vi "Main 2.vi"() -> ()   [LabVIEW 2013]
uses:
  Time_Slot--Control.ctl
  <vilib>/lvdsc/historical/Read Traces (Numeric).vi
  <vilib>/lvdsc/NI_DSC.lvlib
  <vilib>/lvdsc/historical/Read Trace (Numeric).vi
  <userlib>/_OpenG.lib/array/array.llb/Index 1D Array Elements (String)__ogtk.vi
panel:
  in  "Tree":string[](tree)
  out "error out":errorcluster
  out "quality":i32[][](array[numeric])
  in  "options":T1={"interpolate data (F)"=TRUE, "extrapolate to now (F)"=FALSE, "remove data breaks (F)"=TRUE, "interpolation interval (1 s)"=1.0, "maintain trending info (T)"=FALSE} {"interpolation interval (1 s)" min=0.0 format="%0.2f"}
  out "empty?":bool
  out "Argument":string
  in  "Traces":T2(array[cluster])
  out "busy":bool
  out "Array 2":timestamp[](array[timestamp])
  out "Array":timestamp[](array[timestamp])
  out "time (s)":sgl
  out "Children Tags":string[](array[string])
  in  "Presets":u16(ring) items=["Select Preset", "Clear Chart", "Add New Preset"]
  in  "Tab Control":T3(tab)
  in  "Time slots":T4=enum."8 Hours"
  in  "Seek Back Button":bool
  in  "Seek Forward Button":bool
  in  "Display Current":bool
  in  "time interval":T5 {"stop timestamp (now)" format="%<%X\n%x>T"; "start timestamp" format="%<%X\n%x>T"}
  in  "Display Chose Time Slot":bool
  in  "update rate(ms)":i32=10000
  in  "max points per trace (all)":i32=1000
  in  "OK":bool
  out "XY Graph":T6(graph)
  # "Time Window (drop down 1hr 1 day etc)\nchoose channel/s\npresets (inc time window and channels)\nExport to csv.\nLive mode return\nIf you select manual time interval shows that until live mode return button pressed\nwould be nice to have arrows to go back and forth in time."
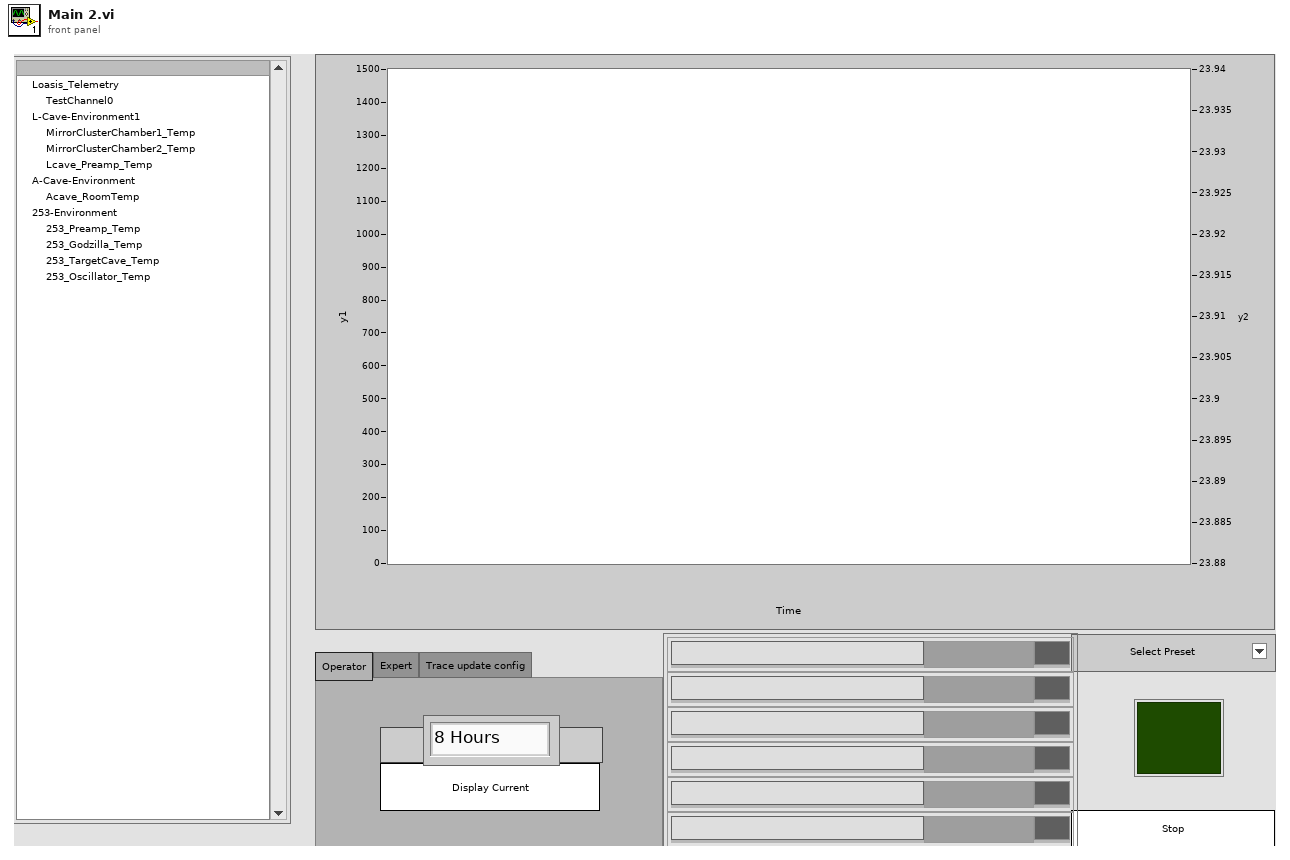
[diagram p1: front panel]
types:
  T1 = cluster{"interpolate data (F)":bool, "extrapolate to now (F)":bool, "remove data breaks (F)":bool, "interpolation interval (1 s)":dbl, "maintain trending info (T)":bool}
  T2 = cluster{"Name":string, "L/R scale":bool, "Color Box":u32}[]
  T3 = enum32{"Operator", "Expert", "Trace update config"}
  T4 = typedef "Time_Slot--Control.ctl" = enum16{"5 Mins", "15 Mins", "30 mins", "1 Hour", "8 Hours", "1 Day", "1 Week", "1 Month", "3 Months", "6 Months", "1 Year", "2 Years"}
  T5 = cluster{"start timestamp":timestamp, "stop timestamp (now)":timestamp}
  T6 = cluster{"timestamps":timestamp[], "data":dbl[]}[]
  T7 = cluster{"Name":string, "L/R scale":bool, "Color Box":u32}
  T8 = enum32{"invalid app kind", "Development System", "Run Time System", "Student Edition", "Embedded LabVIEW", "Evaluation", "Custom"}
  T9 = enum32{"Invalid", "Standard", "Closed", "Hidden", "Minimized", "Maximized"}
  T10 = cluster{"Core":cluster{"Current VI Reference":refnum<vi>, "Close Panel on Exit?":bool}, "options":cluster{"interpolate data (F)":bool, "extrapolate to now (F)":bool, "remove data breaks (F)":bool, "interpolation interval (1 s)":dbl, "maintain trending info (T)":bool}, "time interval":cluster{"start timestamp":timestamp, "stop timestamp (now)":timestamp}, "historical traces":cluster{"timestamps":timestamp[], "data":dbl[]}[], "Trace Names":string[], "max points per trace (all)":i32, "Time slots":T4, "Display Current Enable":bool, "update rate(ms)":i32, "All Traces from DB":string[], "Traces":cluster{"Name":string, "L/R scale":bool, "Color Box":u32}[]}
  T11 = typedef "mysql_authentication.ctl" = cluster{"User":string, "Password":string, "Database":string}
  T12 = cluster{"Port":u16, "IP Address":string, "Authentication":T11}
  T13 = cluster{"Current VI Reference":refnum<vi>, "Close Panel on Exit?":bool}
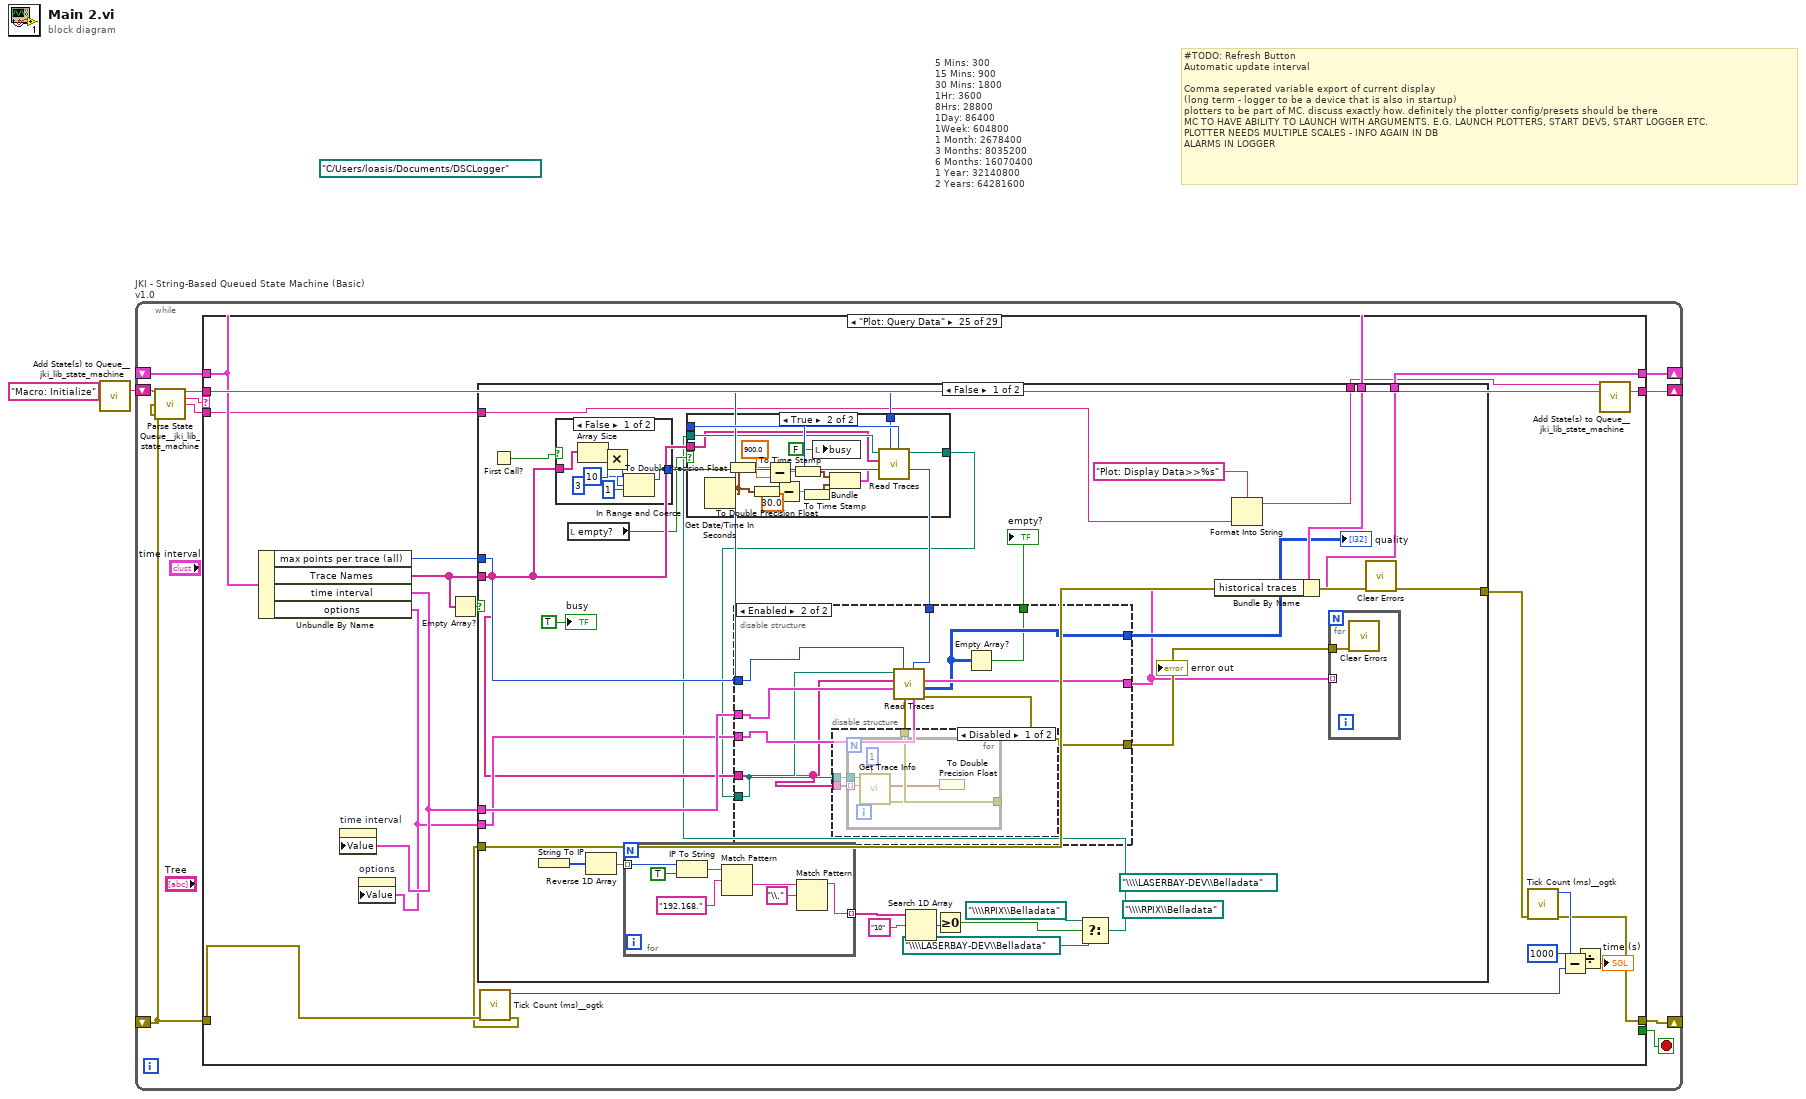
[diagram p0: block diagram]
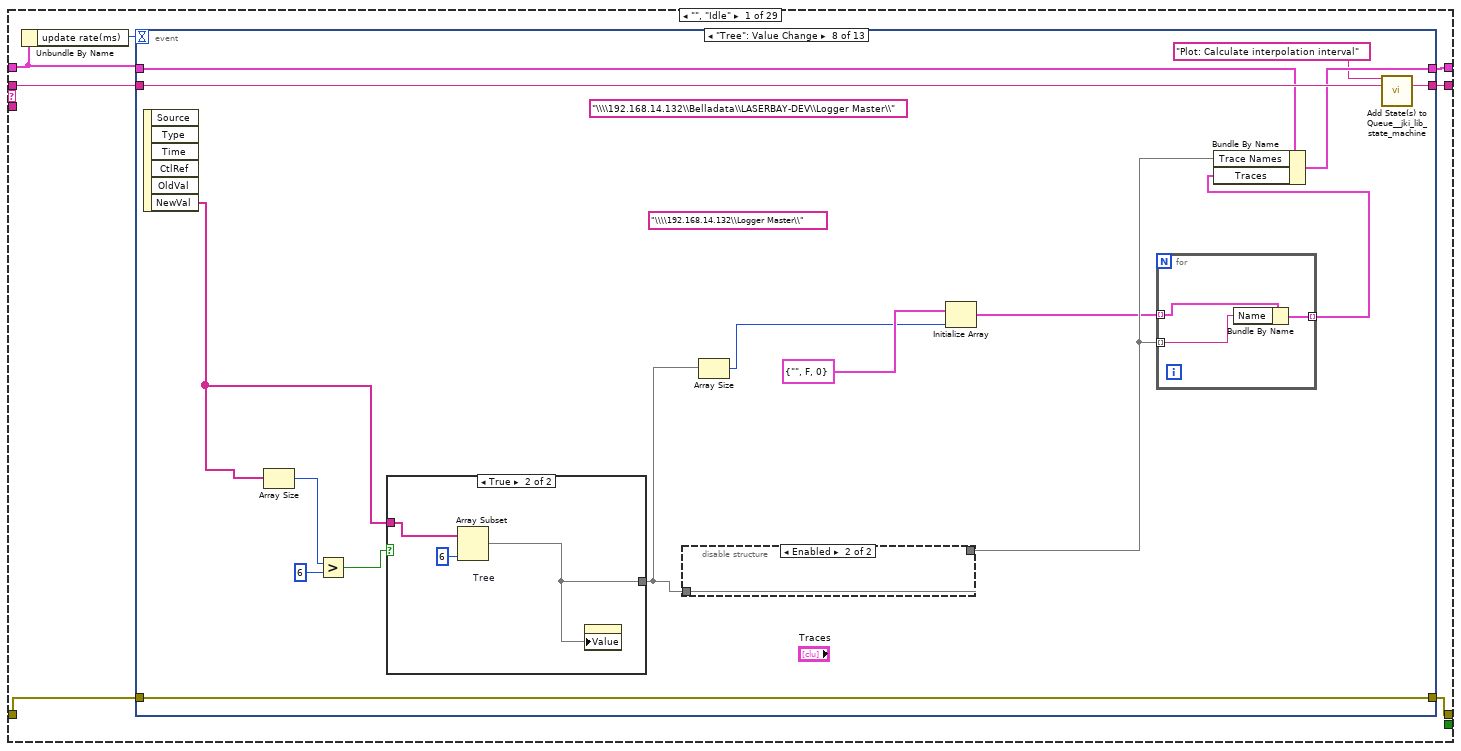
[diagram p2: hidden frame]
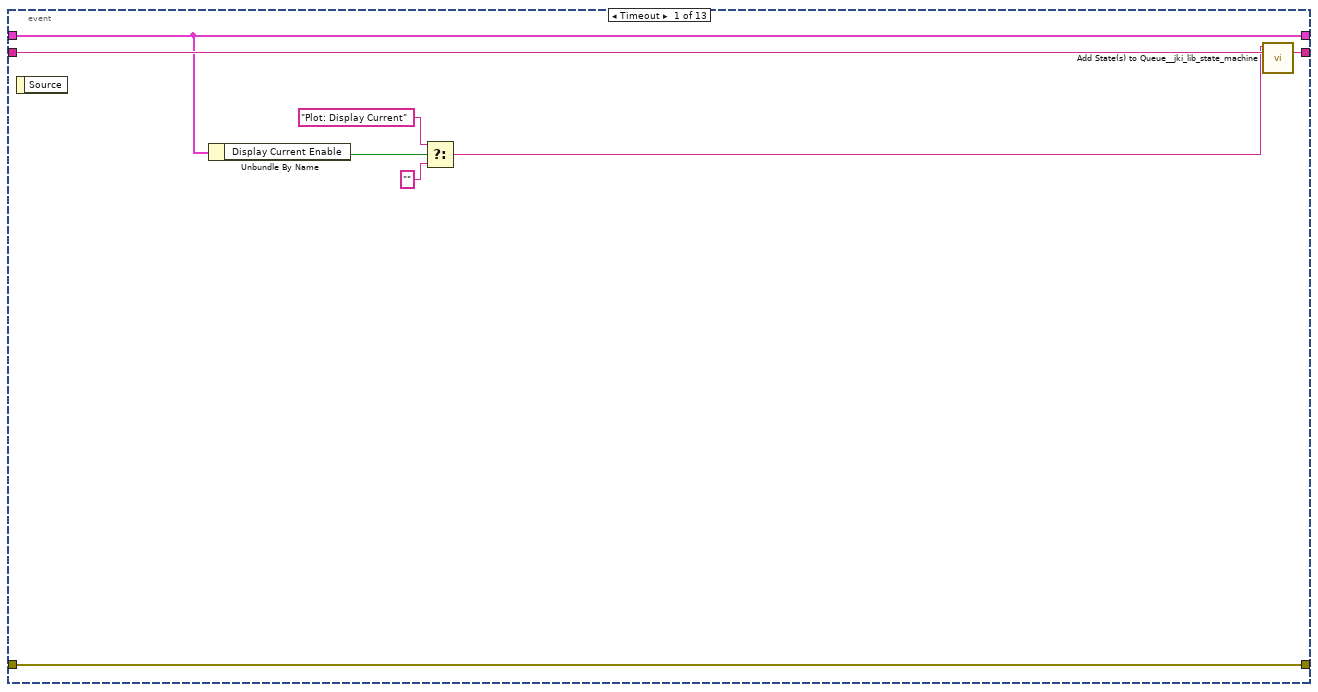
[diagram p3: hidden frame]
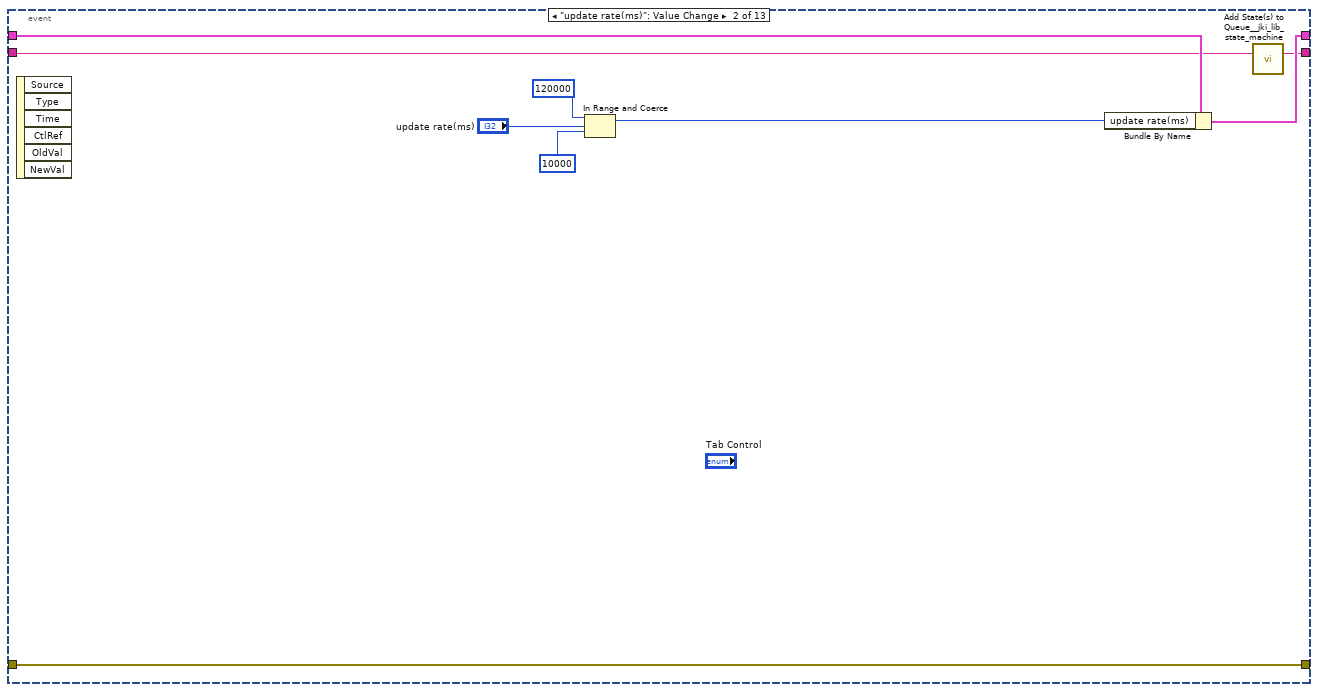
[diagram p4: hidden frame]
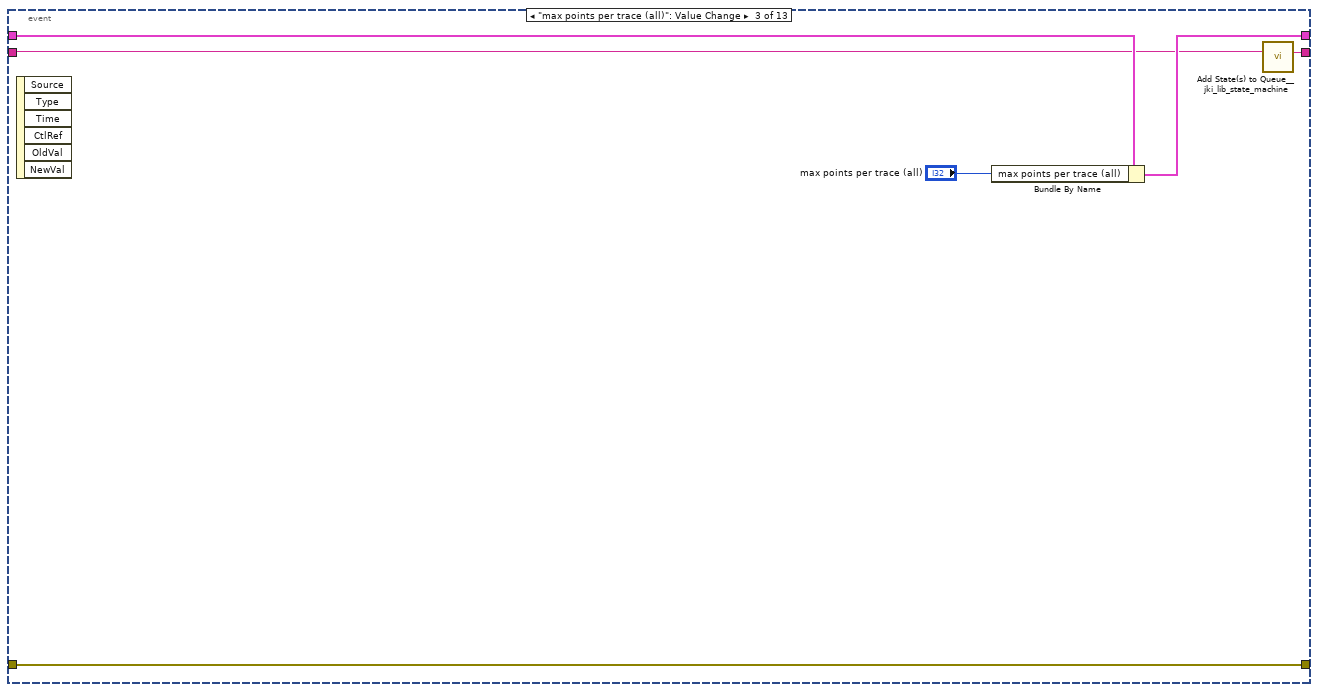
[diagram p5: hidden frame]
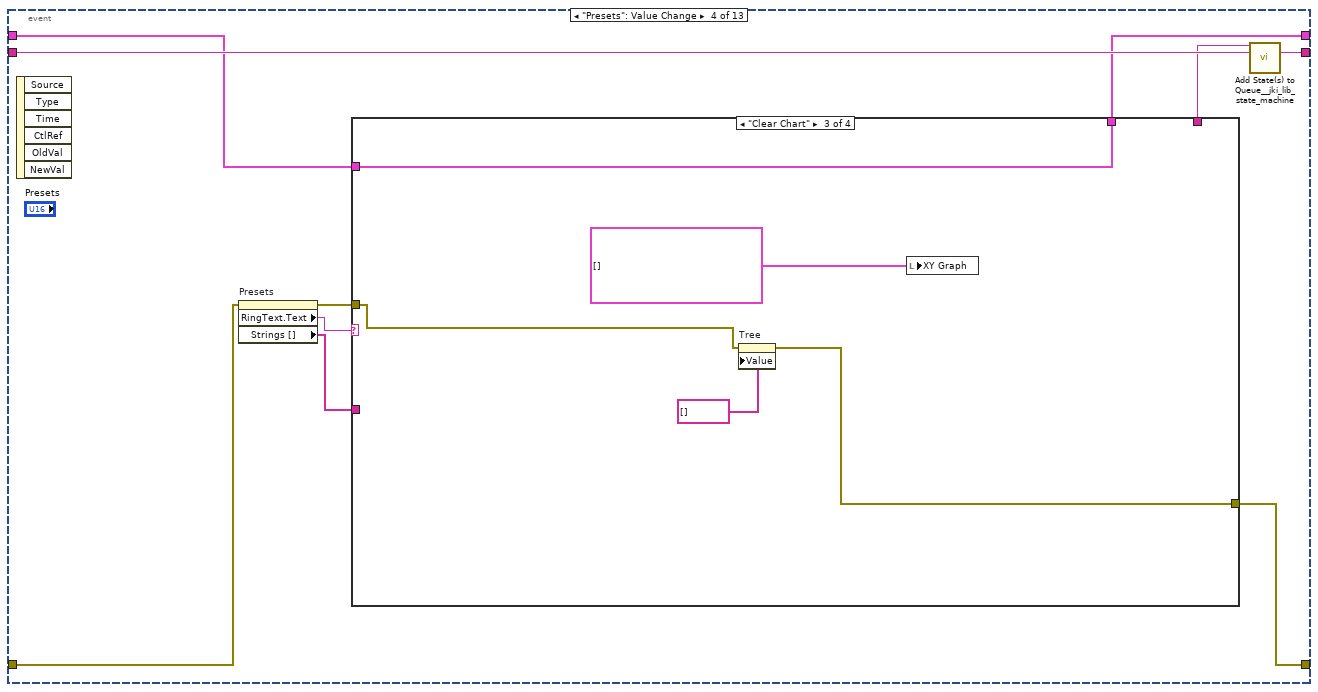
[diagram p6: hidden frame]
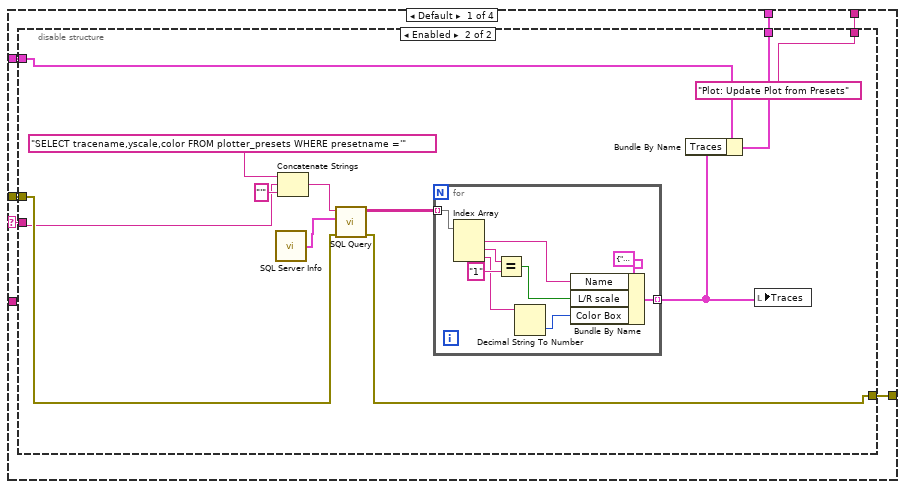
[diagram p7: hidden frame]
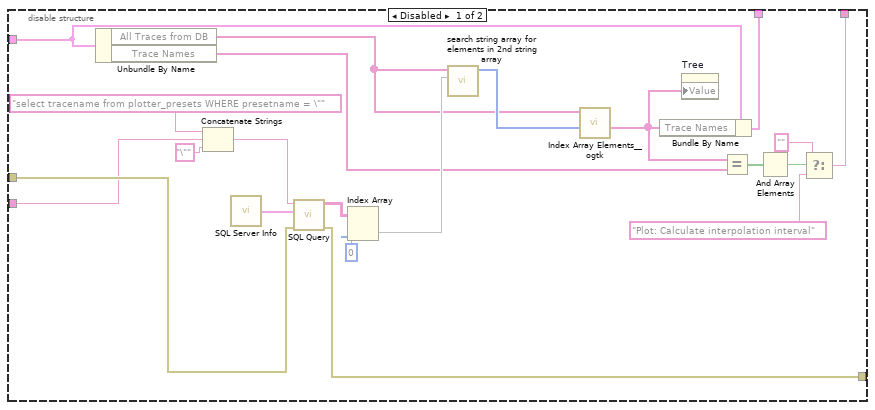
[diagram p8: hidden frame]
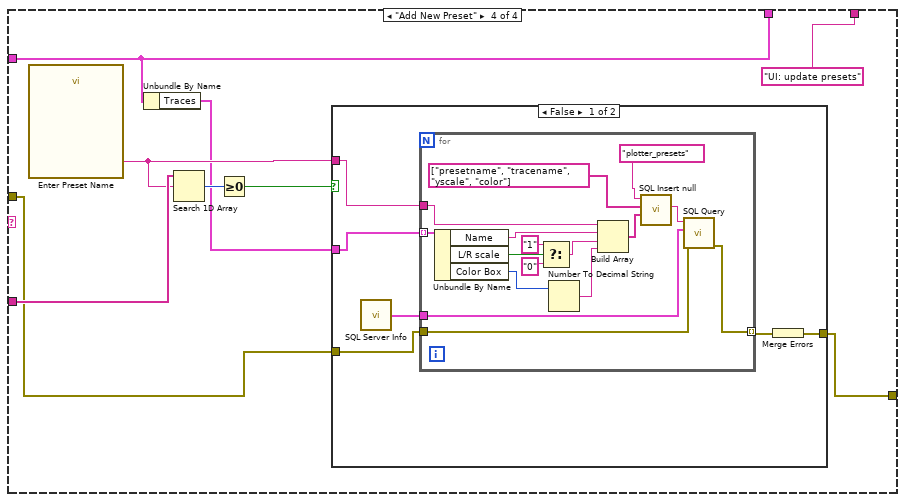
[diagram p10: hidden frame]
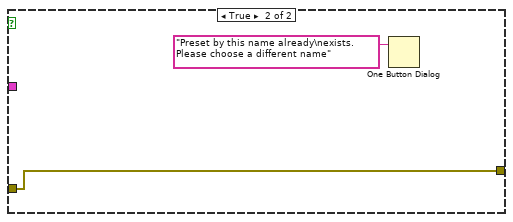
[diagram p11: hidden frame]
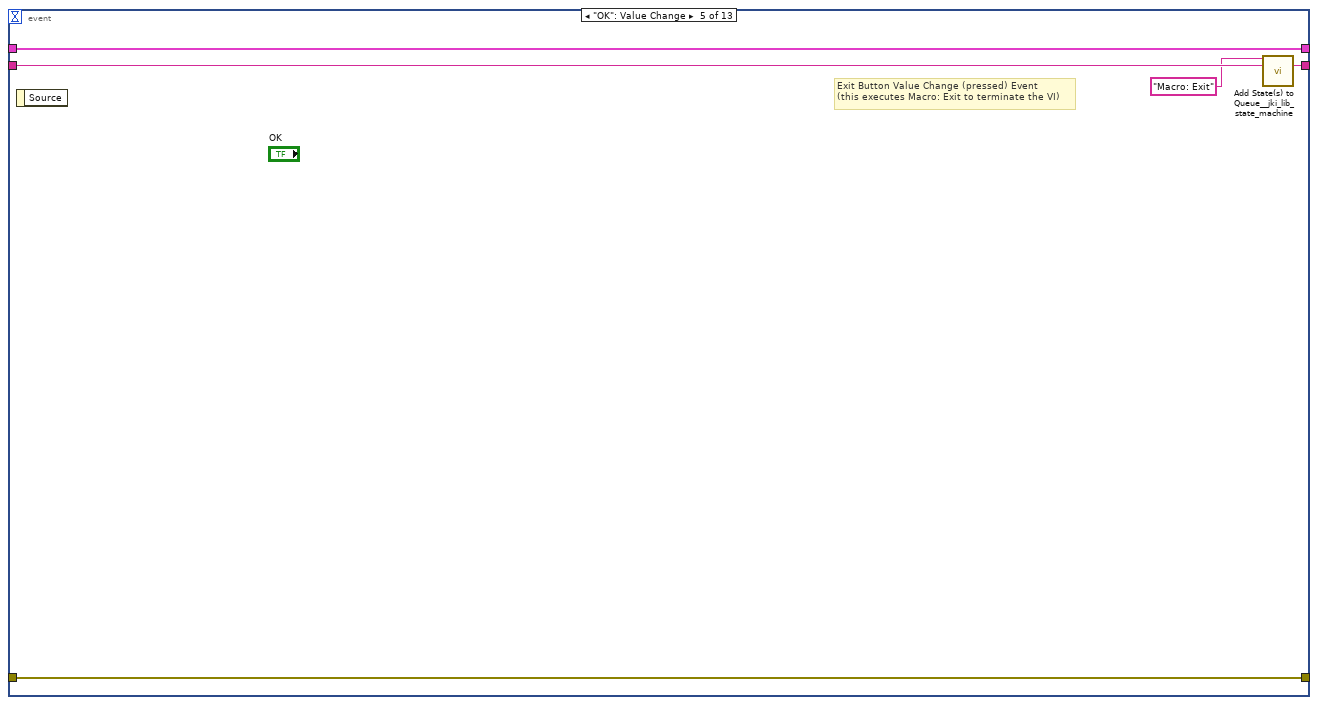
[diagram p12: hidden frame]
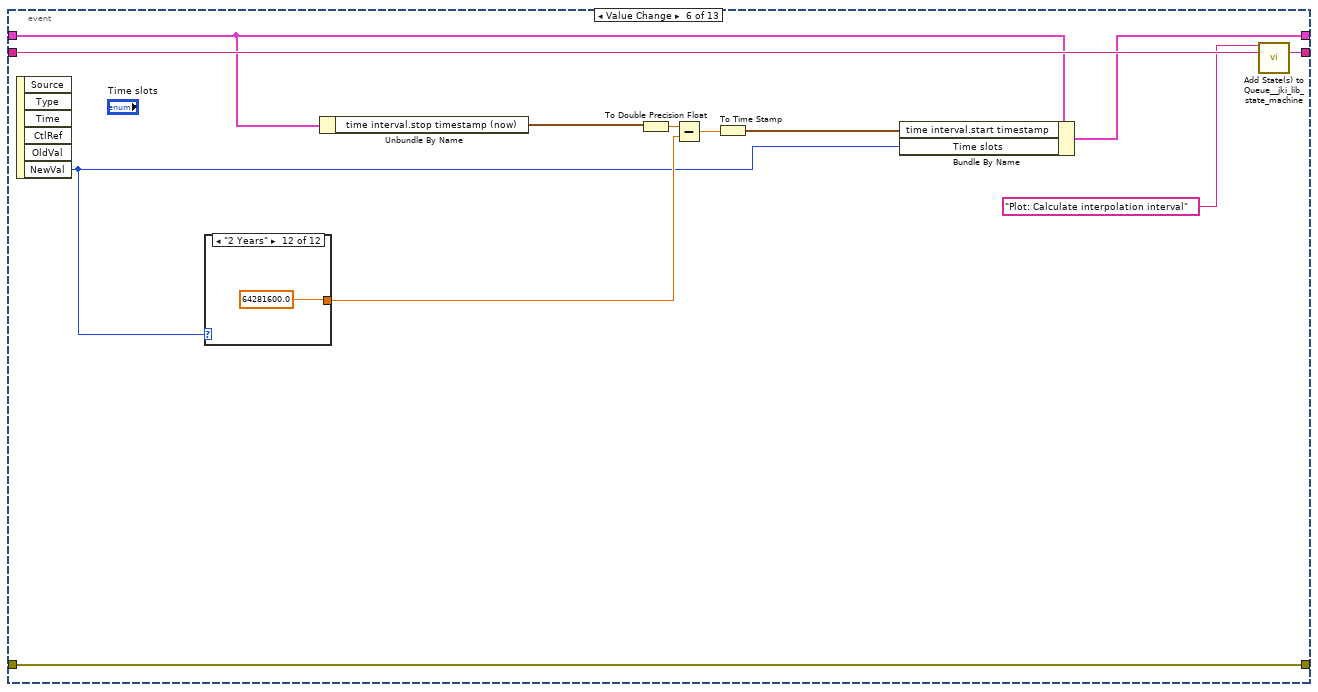
[diagram p13: hidden frame]
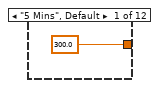
[diagram p14: hidden frame]
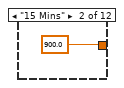
[diagram p15: hidden frame]
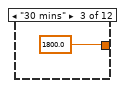
[diagram p16: hidden frame]
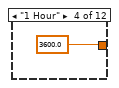
[diagram p17: hidden frame]
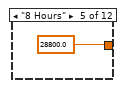
[diagram p18: hidden frame]
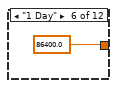
[diagram p19: hidden frame]
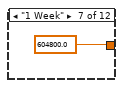
[diagram p20: hidden frame]
diagram:
  (unwired) path "C:/Users/loasis/Documents/DSCLogger" ("Application Directory")
  # "#TODO: Refresh Button\nAutomatic update interval\n\nComma seperated variable export of current display\n(long term - logger to be a device that is also in startup)\nplotters to be part of MC. discuss exactly how. definitely the plotter config/presets should be there\nMC TO HAVE ABILITY TO LAUNCH WITH ARGUMENTS. E.G. LAUNCH PLOTTERS, START DEVS, START LOGGER ETC.\nPLOTTER NEEDS MULTIPLE SCALES - INFO AGAIN IN DB\nALARMS IN LOGGER"
  # "5 Mins: 300\n15 Mins: 900\n30 Mins: 1800\n1Hr: 3600\n8Hrs: 28800\n1Day: 86400\n1Week: 604800\n1 Month: 2678400\n3 Months: 8035200\n6 Months: 16070400 \n1 Year: 32140800\n2 Years: 64281600"
  n1 = call <vilib>:"Add State(s) to Queue__jki_lib_state_machine.vi"("State(s) in (\"\")"="Macro: Initialize") -> ("States Out"=w2:string)  [unwired: 14 in]
  n2 = while "JKI - String-Based Queued State Machine (Basic) v1.0" {
    shift-right: [w5] -> _
    shift-left: _ -> [w4]
    shift-right: [w8] -> _
    shift-left: _ -> [w3]
    shift-right: [w7] -> _
    shift-left: w2 -> [w9]
    stop <- w6 stop-if-true
    n3 = call <vilib>:"Parse State Queue__jki_lib_state_machine.vi"("State Queue"=w9, "Error In (no error)"=w3) -> ("Remaining States"=w11:string, "Current State"=w12:string, "Arguments"=w10:string)  [unwired: 11 in]
    n4 = case shown="\"Plot: Query Data\"" w12 {
      selector: w12 -> [_ _ w346 _ _ _ _ _ _ _ _ _ _ _ _ _ _ _ _ _ _ _ _ _ _ _ _ _ _]
      tunnel: w11 -> [w19 w345 w350 w368 w374 w379 w383 w404 w410 w414 w429 w442 w470 w486 w497 w523 w528 w538 w542 w546 w551 w568 w577 w600 w620 w744 w761 w772 w782]
      tunnel: w10 -> [_ _ _ _ _ _ _ _ _ _ _ _ _ w481 w491 _ _ _ _ _ _ _ _ w587 w601 w738 _ _ _]
      tunnel: w4 -> [w14 w342 w348 w359 w371 w377 w380 _ w405 w411 w427 w440 w472 w484 w493 w520 w525 w535 w539 w543 w548 w564 w573 w593 w616 w742 w759 w770 w777]
      tunnel: [w17 w343 w352 w365 errorcluster {"status"=FALSE, "code"=0, "source"=""} ("error out") w376 w381 w401 w406 w412 w415 w430 w465 w482 w494 w521 w526 w536 w540 w544 w549 w566 w575 w598 w606 w741 w758 w764 w778] -> w8
      tunnel: w3 -> [w16 w343 w351 w365 w370 w376 w381 w401 w407 w412 w416 w431 w466 w483 w495 w521 w526 w536 w540 w544 w549 w566 w575 w598 w610 w741 w758 w765 w774]
      tunnel: [w18 w344 w349 w367 w373 w378 w382 w403 w409 w413 w428 w441 w471 w485 w496 w522 w527 w537 w541 w545 w550 w567 w576 w599 w619 w743 w760 w771 w781] -> w7
      tunnel: [_ _ _ _ _ TRUE _ _ _ _ _ _ _ _ _ _ _ _ _ _ _ _ _ _ _ _ _ _ _] -> w6
      tunnel: [w15 w342 w348 w366 w371 w377 w380 w402 w405 w411 w427 w440 w472 w484 w493 w520 w525 w535 w539 w543 w548 w563 w572 w592 w615 w742 w759 w769 w776] -> w5
      frame "", "Idle" {
        n5 = Unbundle By Name(w14) -> ("update rate(ms)"=w13:i32)
        n6 = event shown="[7] \"Tree\": Value Change" {
          selector: _ -> [_ _ _ _ _ _ _ _ _ _ _ _ _]
          dyn-events: _ -> [_ _ _ _ _ _ _ _ _ _ _ _ _]
          timeout: w13 -> [_ _ _ _ _ _ _ _ _ _ _ _ _]
          tunnel: w19 -> [w27 w28 w37 w47 w145 w155 w172 w188 w207 w250 w283 w312 w341]
          tunnel: [w26 w29 w38 w48 w144 w156 w173 w189 w208 w251 w284 w313 w340] -> w18
          tunnel: w14 -> [w24 w35 w42 w46 w142 w151 w170 w181 w206 w255 w275 w304 w338]
          tunnel: [w25 w30 w39 w49 w143 w157 w174 w190 w209 w248 w285 w314 w339] -> w17
          tunnel: w16 -> [w25 w30 w39 w52 w143 w157 w174 w190 w209 w248 w285 w314 w339]
          tunnel: [w24 w36 w41 w45 w142 w150 w170 w187 w206 w252 w274 w303 w338] -> w15
          event Timeout {
            n7 = event-data() -> ()  [unwired: 1 in, 1 out]
            n8 = Unbundle By Name(w24) -> ("Display Current Enable"=w23:bool)
            n9 = Select(t="Plot: Display Current" ("State(s) in Front (\"\")"), s=w23, f="" ("State(s) in Front (\"\")")) -> (s? t:f=w21:string)
            n10 = call <vilib>:"Add State(s) to Queue__jki_lib_state_machine.vi"("State(s) in Front (\"\")"=w21, "State(s) in (\"\")"=w27) -> ("States Out"=w26:string)  [unwired: 13 in]
          }
          event "update rate(ms)": Value Change {
            n11 = event-data() -> ()  [unwired: 1 in, 6 out]
            n12 = In Range and Coerce(upper limit=120000, x="update rate(ms)", lower limit=10000) -> (coerced(x)=w31:i32)  [unwired: 1 out]
            n13 = Bundle By Name(cluster=w35, "update rate(ms)"=w31) -> (w36:T10)
            n14 = call <vilib>:"Add State(s) to Queue__jki_lib_state_machine.vi"("State(s) in (\"\")"=w28) -> ("States Out"=w29:string)  [unwired: 14 in]
          }
          event "max points per trace (all)": Value Change {
            n15 = event-data() -> ()  [unwired: 1 in, 6 out]
            n16 = Bundle By Name(cluster=w42, "max points per trace (all)"="max points per trace (all)") -> (w41:T10)
            n17 = call <vilib>:"Add State(s) to Queue__jki_lib_state_machine.vi"("State(s) in (\"\")"=w37) -> ("States Out"=w38:string)  [unwired: 14 in]
          }
          event "Presets": Value Change {
            n18 = event-data() -> ()  [unwired: 1 in, 6 out]
            n19 = property on="Presets" class="Ring (strict)"(error in=w52) -> (error out=w50:errorcluster, "RingText.Text"=w51:string, "Strings []"=w43:string[])  [unwired: 1 in, 1 out]
            n20 = case shown="\"Clear Chart\"" w51 {
              selector: w51 -> [w56 _ _ _]
              tunnel: w50 -> [w58 w101 w103 w112]
              tunnel: [w57 w101 w104 w111] -> w49
              tunnel: w46 -> [w55 w102 w107 w110]
              tunnel: [w54 w102 w107 w110] -> w45
              tunnel: [w53 _ _ "UI: update presets" ("t")] -> w44
              tunnel: w43 -> [_ _ _ w116]
              frame Default {
                n21 = disable-structure shown="Enabled" {
                  disable-tunnel: w58 -> [w78 w86]
                  disable-tunnel: [w77 w85] -> w57
                  disable-tunnel: w56 -> [w76 w84]
                  disable-tunnel: w55 -> [w67 w82]
                  disable-tunnel: [w66 w83] -> w54
                  disable-tunnel: [w60 "Plot: Update Plot from Presets" ("t")] -> w53
                  frame Disabled {
                    n22 = Unbundle By Name(w67) -> ("All Traces from DB"=w68:string[], "Trace Names"=w65:string[])
                    n23 = Concatenate Strings("select tracename from plotter_presets WHERE presetname = \"", w76, "\"" ("string")) -> (w74:string)
                    n24 = call "SQL Server Info.vi"() -> ("SQL Server Info"=w79:T12)
                    n25 = call "SQL Query.vi"("error in (no error)"=w78, "SQL Server Info"=w79, "Query"=w74) -> ("error out"=w77:errorcluster, "data"=w72:string[][])  [unwired: 7 in]
                    n26 = Index Array(array=w72, index (col)=0 ("index (row)")) -> (element=w70:string[])  [unwired: 1 in]
                    n27 = call "search string array for elements in 2nd string array.vi"("search for"=w70, "search in"=w68) -> ("Indices of Elements"=w69:i32[])  [unwired: 9 in]
                    n28 = call-poly <userlib>:"Index Array Elements__ogtk.vi"("indices"=w69, "array"=w68) -> ("elements"=w59:string[])  [unwired: 9 in]
                    n29 = Bundle By Name(cluster=w67, "Trace Names"=w59) -> (w66:T10)
                    n30 = property on="Tree" class="Tree (strict)"("Value"=w59) -> ()  [unwired: 2 in, 2 out]
                    n31 = Equal?(x=w59, y=w65) -> (x = y?=w64:bool[])
                    n32 = And Array Elements(Boolean array=w64) -> (logical AND=w63:bool)
                    n33 = Select(t="", s=w63, f="Plot: Calculate interpolation interval") -> (s? t:f=w60:string)
                  }
                  frame Enabled {
                    n34 = call "SQL Server Info.vi"() -> ("SQL Server Info"=w89:T12)
                    n35 = Concatenate Strings("SELECT tracename,yscale,color FROM plotter_presets WHERE presetname ='" ("Query"), w84, "'" ("string")) -> (w91:string)
                    n36 = call "SQL Query.vi"("error in (no error)"=w86, "SQL Server Info"=w89, "Query"=w91) -> ("error out"=w85:errorcluster, "data"=w87:string[][])  [unwired: 7 in]
                    n37 = for {
                      tunnel: w87 -> [w99] mode=indexing
                      tunnel: [w92] -> w81 mode=indexing
                      n38 = Index Array(array=w99) -> (element #1=w98:string, element #2=w97:string, element #3=w93:string)  [unwired: 3 in]
                      n39 = Equal?(x=w97, y="1") -> (x = y?=w95:bool)
                      n40 = Decimal String To Number(string=w93) -> (number=w94:i32)  [unwired: 2 in, 1 out]
                      n41 = Bundle By Name(cluster=T7 {"Name"="", "L/R scale"=FALSE, "Color Box"=0} ("Trace cluster"), "Name"=w98, "L/R scale"=w95, "Color Box"=w94) -> (w92:T7)
                    }
                    n42 = Bundle By Name(cluster=w82, "Traces"=w81) -> (w83:T10)
                    n43 = local write "Traces"(w81) -> ()
                  }
                }
              }
              frame "Select Preset" {
              }
              frame "Clear Chart" {
                n44 = property on="Tree" class="Tree (strict)"(error in=w103, "Value"=string[] [] ("Tree")) -> (error out=w104:errorcluster)  [unwired: 1 in, 1 out]
                n45 = local write "XY Graph"(T6 [] ("XY Graph")) -> ()
              }
              frame "Add New Preset" {
                n46 = call "Enter Preset Name"() -> ("Preset Name"=w113:string)  [unwired: 17 in, 2 out]
                n47 = Unbundle By Name(w110) -> ("Traces"=w109:T2)
                n48 = Search 1D Array(1D array=w116, element=w113) -> (index of element=w115:i32)  [unwired: 1 in]
                n49 = Greater Or Equal To 0?(x=w115) -> (x >= 0?=w114:bool)
                n50 = case shown="False" w114 {
                  tunnel: w109 -> [w121 _]
                  tunnel: w113 -> [w120 _]
                  tunnel: w112 -> [w119 w139]
                  tunnel: [w117 w139] -> w111
                  frame False {
                    n51 = call "SQL Server Info.vi"() -> ("SQL Server Info"=w122:T12)
                    n52 = for {
                      tunnel: w122 -> [w138]
                      tunnel: w121 -> [w130] mode=indexing
                      tunnel: w120 -> [w133]
                      tunnel: w119 -> [w132]
                      tunnel: [w131] -> w118 mode=indexing
                      n53 = Unbundle By Name(w130) -> ("Name"=w129:string, "L/R scale"=w128:bool, "Color Box"=w124:u32)
                      n54 = Select(t="1", s=w128, f="0") -> (s? t:f=w125:string)
                      n55 = Number To Decimal String(number=w124) -> (decimal integer string=w123:string)  [unwired: 1 in]
                      n56 = Build Array(w133, w129, w125, w123) -> (w134:string[])
                      n57 = call "SQL Insert null.vi"("Values"=w134, "Column Names"=string[] ["presetname", "tracename", "yscale", "color"], "Table"="plotter_presets") -> ("Query String"=w137:string)  [unwired: 8 in]
                      n58 = call "SQL Query.vi"("error in (no error)"=w132, "SQL Server Info"=w138, "Query"=w137) -> ("error out"=w131:errorcluster)  [unwired: 7 in, 1 out]
                    }
                    n59 = Merge Errors(w118) -> (w117:errorcluster)
                  }
                  frame True {
                    n60 = One Button Dialog(message="Preset by this name already\nexists. Please choose a different name") -> ()  [unwired: 1 in, 1 out]
                  }
                }
              }
            }
            n61 = call <vilib>:"Add State(s) to Queue__jki_lib_state_machine.vi"("State(s) in Front (\"\")"=w44, "State(s) in (\"\")"=w47) -> ("States Out"=w48:string)  [unwired: 13 in]
          }
          event "OK": Value Change {
            # "Exit Button Value Change (pressed) Event\n(this executes Macro: Exit to terminate the VI)"
            n62 = event-data() -> ()  [unwired: 1 in, 1 out]
            n63 = call <vilib>:"Add State(s) to Queue__jki_lib_state_machine.vi"("State(s) in Front (\"\")"="Macro: Exit", "State(s) in (\"\")"=w145) -> ("States Out"=w144:string)  [unwired: 13 in]
          }
          event Value Change {
            n64 = event-data() -> ("NewVal"=w146:T4)  [unwired: 1 in, 5 out]
            n65 = case shown="\"2 Years\"" w146 {
              tunnel: [300.0 ("y") 900.0 ("y") 1800.0 ("y") 3600.0 ("y") 28800.0 ("y") 86400.0 ("y") 604800.0 ("y") 2678400.0 ("y") 8035200.0 ("y") 16070400.0 ("y") 32140800.0 ("y") 64281600.0 ("y")] -> w152
              frame "5 Mins", Default {
              }
              frame "15 Mins" {
              }
              frame "30 mins" {
              }
              frame "1 Hour" {
              }
              frame "8 Hours" {
              }
              frame "1 Day" {
              }
              frame "1 Week" {
              }
              frame "1 Month" {
              }
              frame "3 Months" {
              }
              frame "6 Months" {
              }
              frame "1 Year" {
              }
              frame "2 Years" {
              }
            }
            n66 = Unbundle By Name(w151) -> ("time interval.stop timestamp (now)"=w153:timestamp)
            n67 = To Double Precision Float(number=w153) -> (double precision float=w154:dbl)
            n68 = Subtract(x=w154, y=w152) -> (x-y=w149:dbl)
            n69 = To Time Stamp(1:w149) -> (0:w148:timestamp)
            n70 = Bundle By Name(cluster=w151, "time interval.start timestamp"=w148, "Time slots"=w146) -> (w150:T10)
            n71 = call <vilib>:"Add State(s) to Queue__jki_lib_state_machine.vi"("State(s) in Front (\"\")"="Plot: Calculate interpolation interval" ("State(s) in Front (\"\")"), "State(s) in (\"\")"=w155) -> ("States Out"=w156:string)  [unwired: 13 in]
          }
          event "Display Current": Value Change {
            n72 = event-data() -> ()  [unwired: 1 in, 6 out]
            n73 = call <vilib>:"Add State(s) to Queue__jki_lib_state_machine.vi"("State(s) in Front (\"\")"="Plot: Display Current" ("State(s) in Front (\"\")"), "State(s) in (\"\")"=w172) -> ("States Out"=w173:string)  [unwired: 13 in]
          }
          event "Tree": Value Change {
            (unwired) "\\\\192.168.14.132\\Belladata\\LASERBAY-DEV\\Logger Master\\"
            (unwired) "\\\\192.168.14.132\\Logger Master\\"
            n74 = event-data() -> ("NewVal"=w182:string[])  [unwired: 1 in, 5 out]
            n75 = Array Size(array=w182) -> (size(s)=w185:i32)
            n76 = Greater?(x=w185, y=6) -> (0:w184:bool)
            n77 = case shown="True" w184 {
              tunnel: w182 -> [w194 w196]
              tunnel: [w194 w195] -> w178
              frame False {
              }
              frame True {
                n78 = Array Subset(array=w196, length=6) -> (w195:string[])  [unwired: 1 in]
                n79 = property on="Tree" class="Tree (strict)"("Value"=w195) -> ()  [unwired: 2 in, 2 out]
              }
            }
            n80 = disable-structure shown="Enabled" {
              disable-tunnel: w178 -> [w199 w202]
              disable-tunnel: [w198 w202] -> w180
              frame Disabled {
                n81 = for {
                  tunnel: w199 -> [w200] mode=indexing
                  tunnel: [w200] -> w198 mode=indexing
                  n82 = Concatenate Strings("\\\\LASERBAY-DEV\\Logger Master\\", w200) -> ()  [unwired: 1 out]
                }
              }
              frame Enabled {
              }
            }
            n83 = Array Size(array=w178) -> (size(s)=w177:i32)
            n84 = Initialize Array(T7 {"Name"="", "L/R scale"=FALSE, "Color Box"=0} ("Trace cluster"), w177) -> (w176:T2)
            n85 = for {
              tunnel: w180 -> [w192] mode=indexing
              tunnel: w176 -> [w193] mode=indexing
              tunnel: [w191] -> w175 mode=indexing
              n86 = Bundle By Name(cluster=w193, "Name"=w192) -> (w191:T7)
            }
            n87 = Bundle By Name(cluster=w181, "Trace Names"=w180, "Traces"=w175) -> (w187:T10)
            n88 = call <vilib>:"Add State(s) to Queue__jki_lib_state_machine.vi"("State(s) in Front (\"\")"="Plot: Calculate interpolation interval" ("State(s) in Front (\"\")"), "State(s) in (\"\")"=w188) -> ("States Out"=w189:string)  [unwired: 13 in]
          }
          event "Traces": Value Change {
            n89 = event-data() -> ("OldVal"=w205:T2, "NewVal"=w204:T2)  [unwired: 1 in, 4 out]
            n90 = for {
              tunnel: w205 -> [w222] mode=indexing
              tunnel: w204 -> [w221] mode=indexing
              tunnel: w204 -> [w213]
              i -> [w212]
              n91 = Unbundle By Name(w221) -> ("Name"=w215:string, "L/R scale"=w219:bool, "Color Box"=w218:u32)
              n92 = Unbundle By Name(w222) -> ("Name"=w216:string, "L/R scale"=w220:bool, "Color Box"=w217:u32)
              n93 = Equal?(x=w217, y=w218) -> (x = y?=w210:bool)
              n94 = Equal?(x=w220, y=w219) -> (x = y?=w214:bool)
              n95 = Equal?(x=w216, y=w215) -> (x = y?=w211:bool)
              n96 = case shown="True" w211 {
                tunnel: w214 -> [_ w226]
                tunnel: w213 -> [_ w225]
                tunnel: w212 -> [_ w224]
                tunnel: w210 -> [_ w223]
                frame False {
                }
                frame True {
                  n97 = stacked-sequence {
                    tunnel: w226 -> [w229 _]
                    tunnel: w225 -> [w228 w240]
                    tunnel: w224 -> [w227 w239]
                    tunnel: w223 -> [_ w241]
                    frame #0 {
                      n98 = case shown="False" w229 {
                        tunnel: w228 -> [w237 _]
                        tunnel: w227 -> [w231 _]
                        frame False {
                          (unwired) u8 2 ("Y Scale.Scale Fit")
                          n99 = Index Array(array=w237, index=w231) -> (element=w236:T7)
                          n100 = Unbundle By Name(w236) -> ("L/R scale"=w235:bool)
                          n101 = To Unsigned Long Integer(number=w231) -> (unsigned 32bit integer=w230:u32)
                          n102 = Select(t=u32 1 ("f"), s=w235, f=u32 0) -> (s? t:f=w233:u32)
                          n103 = control-ref of="XY Graph"() -> (w238:refnum<vi>)
                          n104 = property class="XYGraph (strict)"(reference=w238, "Active Plot"=w230, "Plot.YScaleIdx"=w233) -> ()  [unwired: 1 in, 2 out]
                        }
                        frame True {
                        }
                      }
                    }
                    frame #1 {
                      n105 = case shown="False" w241 {
                        tunnel: w240 -> [w244 _]
                        tunnel: w239 -> [w243 _]
                        frame False {
                          n106 = Index Array(array=w244, index=w243) -> (element=w246:T7)
                          n107 = Unbundle By Name(w246) -> ("Color Box"=w242:u32)
                          n108 = To Unsigned Long Integer(number=w243) -> (unsigned 32bit integer=w245:u32)
                          n109 = control-ref of="XY Graph"() -> (w247:refnum<vi>)
                          n110 = property class="XYGraph (strict)"(reference=w247, "Active Plot"=w245, "Plot.Plot Color"=w242) -> ()  [unwired: 1 in, 2 out]
                        }
                        frame True {
                        }
                      }
                    }
                  }
                }
              }
            }
            n111 = call <vilib>:"Add State(s) to Queue__jki_lib_state_machine.vi"("State(s) in Front (\"\")"="Plot: Display Data" ("State(s) in Front (\"\")"), "State(s) in (\"\")"=w207) -> ("States Out"=w208:string)  [unwired: 13 in]
          }
          event "Display Chose Time Slot": Value Change {
            n112 = event-data() -> ()  [unwired: 1 in, 6 out]
            n113 = property on="time interval" class="Clust (strict)"() -> ("Value"=w261:T5)  [unwired: 2 in, 2 out]
            n114 = Unbundle By Name(w261) -> ("start timestamp"=w254:timestamp, "stop timestamp (now)"=w253:timestamp)
            n115 = To Double Precision Float(number=w254) -> (double precision float=w259:dbl)
            n116 = To Double Precision Float(number=w253) -> (double precision float=w260:dbl)
            n117 = Subtract(x=w259, y=w260) -> (x-y=w258:dbl)
            n118 = Greater?(x=w258, y=60.0) -> (0:w256:bool)
            n119 = case shown="True" w256 {
              tunnel: w255 -> [w263 w268]
              tunnel: w254 -> [_ w267]
              tunnel: w253 -> [_ w266]
              tunnel: [w263 w265] -> w252
              tunnel: ["" "Plot: Calculate interpolation interval" ("State(s) in Front (\"\")")] -> w249
              frame False {
              }
              frame True {
                n120 = Bundle By Name(cluster=w268, "time interval.start timestamp"=w267, "time interval.stop timestamp (now)"=w266) -> (w265:T10)
              }
            }
            n121 = call <vilib>:"Add State(s) to Queue__jki_lib_state_machine.vi"("State(s) in Front (\"\")"=w249, "State(s) in (\"\")"=w250) -> ("States Out"=w251:string)  [unwired: 13 in]
          }
          event "Seek Back Button": Value Change {
            n122 = event-data() -> ()  [unwired: 1 in, 6 out]
            n123 = Unbundle By Name(w275) -> ("Time slots"=w281:T4)
            n124 = case shown="\"15 Mins\"" w281 {
              tunnel: [300.0 ("y") 900.0 ("y") 1800.0 ("y") 3600.0 ("y") 28800.0 ("y") 86400.0 ("y") 604800.0 ("y") 2678400.0 ("y") 8035200.0 ("y") 16070400.0 ("y") 32140800.0 ("y") 64281600.0 ("y")] -> w276
              frame "5 Mins", Default {
              }
              frame "15 Mins" {
              }
              frame "30 mins" {
              }
              frame "1 Hour" {
              }
              frame "8 Hours" {
              }
              frame "1 Day" {
              }
              frame "1 Week" {
              }
              frame "1 Month" {
              }
              frame "3 Months" {
              }
              frame "6 Months" {
              }
              frame "1 Year" {
              }
              frame "2 Years" {
              }
            }
            n125 = Unbundle By Name(w275) -> ("time interval.start timestamp"=w279:timestamp, "time interval.stop timestamp (now)"=w277:timestamp)
            n126 = To Double Precision Float(number=w279) -> (double precision float=w280:dbl)
            n127 = To Double Precision Float(number=w277) -> (double precision float=w278:dbl)
            n128 = Subtract(x=w280, y=w276) -> (x-y=w273:dbl)
            n129 = Subtract(x=w278, y=w276) -> (x-y=w270:dbl)
            n130 = To Time Stamp(1:w273) -> (0:w272:timestamp)
            n131 = To Time Stamp(1:w270) -> (0:w271:timestamp)
            n132 = Bundle By Name(cluster=w275, "time interval.start timestamp"=w272, "time interval.stop timestamp (now)"=w271, "Display Current Enable"=FALSE) -> (w274:T10)
            n133 = call <vilib>:"Add State(s) to Queue__jki_lib_state_machine.vi"("State(s) in Front (\"\")"="Plot: Calculate interpolation interval" ("State(s) in Front (\"\")"), "State(s) in (\"\")"=w283) -> ("States Out"=w284:string)  [unwired: 13 in]
          }
          event "Seek Forward Button": Value Change {
            n134 = event-data() -> ()  [unwired: 1 in, 6 out]
            n135 = Unbundle By Name(w304) -> ("Time slots"=w310:T4)
            n136 = case shown="\"2 Years\"" w310 {
              tunnel: [300.0 ("y") 900.0 ("y") 1800.0 ("y") 3600.0 ("y") 28800.0 ("y") 86400.0 ("y") 604800.0 ("y") 2678400.0 ("y") 8035200.0 ("y") 16070400.0 ("y") 32140800.0 ("y") 64281600.0 ("y")] -> w305
              frame "5 Mins", Default {
              }
              frame "15 Mins" {
              }
              frame "30 mins" {
              }
              frame "1 Hour" {
              }
              frame "8 Hours" {
              }
              frame "1 Day" {
              }
              frame "1 Week" {
              }
              frame "1 Month" {
              }
              frame "3 Months" {
              }
              frame "6 Months" {
              }
              frame "1 Year" {
              }
              frame "2 Years" {
              }
            }
            n137 = Unbundle By Name(w304) -> ("time interval.start timestamp"=w308:timestamp, "time interval.stop timestamp (now)"=w306:timestamp)
            n138 = Get Date/Time In Seconds() -> (seconds since 1Jan1904=w301:timestamp)
            n139 = To Double Precision Float(number=w301) -> (double precision float=w299:dbl)
            n140 = To Double Precision Float(number=w308) -> (double precision float=w309:dbl)
            n141 = To Double Precision Float(number=w306) -> (double precision float=w307:dbl)
            n142 = Add(x=w309, y=w305) -> (x+y=w302:dbl)
            n143 = Add(x=w307, y=w305) -> (x+y=w300:dbl)
            n144 = Greater?(x=w300, y=w299) -> (0:w298:bool)
            n145 = case shown="True" w298 {
              tunnel: ["Plot: Calculate interpolation interval" ("State(s) in Front (\"\")") "Plot: Display Current" ("State(s) in Front (\"\")")] -> w311
              tunnel: w304 -> [w320 w322]
              tunnel: [w319 w322] -> w303
              tunnel: w302 -> [w318 _]
              tunnel: w300 -> [w315 _]
              frame False {
                n146 = To Time Stamp(1:w318) -> (0:w317:timestamp)
                n147 = To Time Stamp(1:w315) -> (0:w316:timestamp)
                n148 = Bundle By Name(cluster=w320, "time interval.start timestamp"=w317, "time interval.stop timestamp (now)"=w316) -> (w319:T10)
              }
              frame True {
              }
            }
            n149 = call <vilib>:"Add State(s) to Queue__jki_lib_state_machine.vi"("State(s) in Front (\"\")"=w311, "State(s) in (\"\")"=w312) -> ("States Out"=w313:string)  [unwired: 13 in]
          }
          event Panel Close? {
            # "Discard the event because we'll close the front panel ourselves in Macro: Exit"
            # "Close Panel button (pressed) Event\n(this executes Macro: Exit to terminate the VI)"
            n150 = event-data() -> ()  [unwired: 1 in, 1 out]
            n151 = event-data("Discard?"=TRUE) -> ()  [unwired: 1 in, 1 out]
            n152 = call <vilib>:"Add State(s) to Queue__jki_lib_state_machine.vi"("State(s) in Front (\"\")"="Macro: Exit", "State(s) in (\"\")"=w341) -> ("States Out"=w340:string)  [unwired: 13 in]
          }
        }
      }
      frame "---------- Core ----------" {
        # "Do not put any code in this frame.\n(it is a separator no-op)"
        n153 = call <vilib>:"Add State(s) to Queue__jki_lib_state_machine.vi"("State(s) in (\"\")"=w345) -> ("States Out"=w344:string)  [unwired: 14 in]
      }
      frame Default {
        w355 = 42 items=["No error", "Argument error", "Memory is full", "Out of zone", "End of file", "File already open", "Generic file I/O error", "File not found", "File permission error", "Disk is full", "Duplicate path", "Too many files open", "System feature not enabled", "Resource file not found", "Cannot add resource", "Resource not found", "Image not found", "Image memory error", "Pen does not exist", "Config type invalid", "Config token not found", "Config parse error", "Config memory error", "Bad external code format", "Bad external code offset", "External code not present", "Null window", "Destroy window error", "Null menu", "Print aborted", "Bad print record", "Print driver error", "Windows error during printing", "Memory error during printing", "Print dialog error", "Generic print error", "Invalid device refnum", "Device not found", "Device parameter error", "Device unit error", "Cannot open device", "Device call aborted", "Generic error", "Cancelled by user", "Object ID too low", "Object ID too high", "Object not in heap", "Unknown heap", "Unknown object (invalid DefProc)", "Unknown object (DefProc not in table)", "Message out of range", "Invalid (null) method", "Unknown message", "Manager call not supported", "Bad address", "Network operation in progress", "Network operation timed out", "Connection is busy", "Network attribute not supported", "Network error", "Address in use", "System out of memory", "Connection aborted", "Connection refused", "Not connected", "Already connected", "Connection closed", "Initialization error (interapplication manager)", "Bad occurrence", "Wait on unbound occurrence handler", "Occurrence queue overflow", "Datalog type conflict", "Unused", "Unrecognized type (interapplication manager)", "Memory corrupt", "Failed to make temporary DLL", "Old CIN version", "Drag socket not found", "Failed to load drop-object", "Failed to register OLE object", "Failed to release OLE object", "Format specifier type mismatch", "Unknown format specifier", "Too few format specifiers", "Too many format specifiers", "Scan failed", "Newer CIN version", "Error converting to variant", "Runtime menu error", "Password tampered", "Variant attribute not found", "Incompatible variant data type", "Event data is not available", "Event Store is not present", "Occurrence is not found", "Event Queue is not created", "Event info is not available", "Refnum passed is NULL", "Error retrieving Class GUID", "Error retrieving CoClass GUID", "Error retrieving TypeLib GUID.", "Bad built application magic bytes.", "Specific driver is different from the specific driver associated with the Logical Name.", "There is no session opened to the class driver.", "Max Error", "MAX - Error with config objects", "MAX - Error loading configuration", "MAX - Group not supported"]
        # "Current State"
        # "Do not delete, rename, or modify this frame.\n(this is used to capture unhandled states and typos)"
        # "Handle mistyped state name (developer tool)"
        n154 = Format Into String(format string="Software Exception: Unhandled State \"%s\"." ("message"), error in=w351, w346) -> (resulting string=w354:string, error out=w353:errorcluster)  [unwired: 1 in]
        n155 = call <vilib>:"Error Cluster From Error Code.vi"("show call chain? (False)"=TRUE, "error in (no error)"=w353, "error message (\"\")"=w354, "error code (0)"=w355) -> ("error out"=w352:errorcluster)  [unwired: 5 in]
        n156 = call <vilib>:"Add State(s) to Queue__jki_lib_state_machine.vi"("State(s) in (\"\")"=w350) -> ("States Out"=w349:string)  [unwired: 14 in]
      }
      frame "Initialize Core Data" {
        # "Do not delete, rename, or modify this frame.\n(this is used to determine panel behavior on exit)"
        # "originally closed?"
        # "exe?"
        # "If panel starts closed or is an EXE, then close it when we exit"
        n157 = property class="VI"() -> ("Front Panel.Open"=w364:bool)  [unwired: 2 in, 2 out]
        n158 = property class="App"() -> ("App.Kind"=w363:T8)  [unwired: 2 in, 2 out]
        n159 = control-ref of="Current VI Reference"() -> (w357:refnum<vi>)
        n160 = Not(x=w364) -> (.not. x?=w361:bool)
        n161 = Equal?(x=w363, y=T8."Run Time System" ("Application:Kind")) -> (x = y?=w360:bool)
        n162 = Or(x=w361, y=w360) -> (x .or. y?=w358:bool)
        n163 = Bundle By Name(cluster=w359, "Core.Current VI Reference"=w357, "Core.Close Panel on Exit?"=w358) -> (w366:T10)
        n164 = call <vilib>:"Add State(s) to Queue__jki_lib_state_machine.vi"("State(s) in (\"\")"=w368) -> ("States Out"=w367:string)  [unwired: 14 in]
      }
      frame "Error Handler" {
        # "Unhandled Error -- Display it"
        # "Handle any errors here.\nYou can also output any states to clean-up after errors occur"
        # "Clear error"
        n165 = call <vilib>:"General Error Handler.vi"("error in (no error)"=w370) -> ()  [unwired: 10 in, 5 out]
        n166 = call <vilib>:"Add State(s) to Queue__jki_lib_state_machine.vi"("State(s) in Front (\"\")"="/* Post Error States", "State(s) in (\"\")"=w374) -> ("States Out"=w373:string)  [unwired: 13 in]
      }
      frame "Exit" {
        # "Do not put any code in this frame.\n(No errors that occur here will be handled.)"
        n167 = call <vilib>:"Add State(s) to Queue__jki_lib_state_machine.vi"("State(s) in (\"\")"=w379) -> ("States Out"=w378:string)  [unwired: 14 in]
      }
      frame "---------- Data ----------" {
        # "Do not put any code in this frame.\n(It is a separator no-op. You can make a copy of this frame to create a new Data frame)"
        n168 = call <vilib>:"Add State(s) to Queue__jki_lib_state_machine.vi"("State(s) in (\"\")"=w383) -> ("States Out"=w382:string)  [unwired: 14 in]
      }
      frame "Data: Initialize" {
        w384 = T2 []  # Traces
        w385 = string[] []  # All Traces from DB
        w386 = 1000  # max points per trace (all)
        w387 = 60000  # update rate(ms)
        w388 = T5 {"start timestamp"=timestamp(0 s since 1904-01-01), "stop timestamp (now)"=timestamp(0 s since 1904-01-01)}  # time interval
        w389 = TRUE  # Display Current Enable
        w390 = Time_Slot--Control."8 Hours"  # Time slots
        w397 = string[] []  # Trace Names
        w398 = T6 []  # historical traces
        w400 = T13 {"Current VI Reference"=refnum, "Close Panel on Exit?"=FALSE}  # Core
        # "8 Hrs"
        n169 = Get Date/Time In Seconds() -> (seconds since 1Jan1904=w393:timestamp)
        n170 = To Double Precision Float(number=w393) -> (double precision float=w395:dbl)
        n171 = Subtract(x=w395, y=28800.0) -> (x-y=w394:dbl)
        n172 = To Time Stamp(1:w394) -> (0:w391:timestamp)
        n173 = Bundle By Name(cluster=w388, "stop timestamp (now)"=w393, "start timestamp"=w391) -> (w396:T5)
        n174 = property on="Time slots" class="Enum (strict)"("Value"=w390) -> ()  [unwired: 2 in, 2 out]
        n175 = Bundle("Core"=w400, "options"="options", "time interval"=w396, "historical traces"=w398, "Trace Names"=w397, "max points per trace (all)"=w386, "Time slots"=w390, "Display Current Enable"=w389, "update rate(ms)"=w387, "All Traces from DB"=w385, "Traces"=w384) -> (w402:T10)  [unwired: 1 in]
        n176 = call <vilib>:"Add State(s) to Queue__jki_lib_state_machine.vi"("State(s) in (\"\")"=w404) -> ("States Out"=w403:string)  [unwired: 14 in]
      }
      frame "Data: Cleanup" {
        # "Cleanup any data and references, here.\n(this is called automatically, by the Macro: Exit)"
        n177 = Unbundle By Name(w405) -> ("Core.Current VI Reference"=w408:refnum<vi>)
        n178 = Close Reference(reference=w408, error in (no error)=w407) -> (error out=w406:errorcluster)
        n179 = call <vilib>:"Add State(s) to Queue__jki_lib_state_machine.vi"("State(s) in (\"\")"=w410) -> ("States Out"=w409:string)  [unwired: 14 in]
      }
      frame "---------- UI ----------" {
        # "Do not put any code in this frame.\n(It is a separator no-op. You can make a copy of this frame to create a new UI frame)"
        n180 = call <vilib>:"Add State(s) to Queue__jki_lib_state_machine.vi"("State(s) in (\"\")"=w414) -> ("States Out"=w413:string)  [unwired: 14 in]
      }
      frame "UI: update presets" {
        # "Do not put any code in this frame.\n(It is a separator no-op. You can make a copy of this frame to create a new UI frame)"
        n181 = call "SQL Server Info.vi"() -> ("SQL Server Info"=w424:T12)
        n182 = call "SQL Query.vi"("error in (no error)"=w416, "SQL Server Info"=w424, "Query"="SELECT DISTINCT presetname FROM plotter_presets") -> ("error out"=w417:errorcluster, "data"=w426:string[][])  [unwired: 7 in]
        n183 = Index Array(array=w426, index (col)=0 ("disabled index (col)")) -> (element=w420:string[])  [unwired: 1 in]
        n184 = Insert Into Array(array=string[] ["Select Preset", "Clear Chart", "Add New Preset"], index=2, new element=w420) -> (w419:string[])
        n185 = property on="Presets" class="Ring (strict)"(error in=w417, "Strings []"=w419, "Value"=0) -> (error out=w415:errorcluster)  [unwired: 1 in, 1 out]
        n186 = call <vilib>:"Add State(s) to Queue__jki_lib_state_machine.vi"("State(s) in (\"\")"=w429) -> ("States Out"=w428:string)  [unwired: 14 in]
      }
      frame "UI: Initialize" {
        # "Initialize the User Interface, here.\n(this is called automatically, by the Macro: Init)"
        n187 = invoke on="Tree" class="Tree (strict)" method="Reinit To Default"() -> (error out=w432:errorcluster)  [unwired: 3 in, 2 out]
        n188 = call "SQL Server Info.vi"() -> ("SQL Server Info"=w439:T12)
        n189 = call "SQL Query.vi"("error in (no error)"=w431, "SQL Server Info"=w439, "Query"="SELECT DISTINCT channel_group FROM logger") -> ("error out"=w430:errorcluster, "data"=w434:string[][])  [unwired: 7 in]
        n190 = invoke on="Tree" class="Tree (strict)" method="Edit Tree Items.Delete"(error in=w432, "Delete Children"=TRUE ("Delete Children?")) -> (error out=w438:errorcluster)  [unwired: 3 in, 4 out]
        n191 = Index Array(array=w434, index (col)=0 ("disabled index (col)")) -> (element=w436:string[])  [unwired: 1 in]
        n192 = for {
          tunnel: w436 -> [w444] mode=indexing
          tunnel: w438 -> [w450]
          tunnel: w439 -> [w449]
          n193 = invoke on="Tree" class="Tree (strict)" method="Edit Tree Items.Add Item"(error in=w450, "Child Position"=-1 ("Child Posn"), "Left Cell"=w444, "Child Only?"=FALSE) -> (error out=w445:errorcluster)  [unwired: 5 in, 8 out]
          n194 = Concatenate Strings("SELECT device,variable,alias FROM logger WHERE channel_group ='" ("Query"), w444, "'" ("string")) -> (w446:string)
          n195 = call "SQL Query.vi"("error in (no error)"=w445, "SQL Server Info"=w449, "Query"=w446) -> ("data"=w443:string[][])  [unwired: 7 in, 1 out]
          n196 = for {
            tunnel: w444 -> [w462]
            tunnel: w443 -> [w461] mode=indexing
            n197 = Index Array(array=w461) -> (element #1=w453:string, element #2=w455:string, element #3=w457:string)  [unwired: 3 in]
            n198 = Empty String/Path?(string/path=w457) -> (empty?=w460:bool)
            n199 = Concatenate Strings(w453, " " ("string"), w455) -> (w456:string)
            n200 = Select(t=w456, s=w460, f=w457) -> (s? t:f=w458:string)
            n201 = invoke on="Tree" class="Tree (strict)" method="Edit Tree Items.Add Item"("Parent Tag"=w462, "Left Cell"=w458, "Child Tag"=w458, "Child Only?"=TRUE) -> ()  [unwired: 5 in, 9 out]
          }
        }
        n202 = call <vilib>:"Add State(s) to Queue__jki_lib_state_machine.vi"("State(s) in (\"\")"=w442) -> ("States Out"=w441:string)  [unwired: 14 in]
      }
      frame "UI: Get Tree Items" {
        n203 = control-ref of="Tree"() -> (w469:refnum<vi>)
        n204 = call "getchildren.vi"("Tree Reference In"=w469) -> ("Children Tags"=w468:string[], "Tree Reference Out"=w467:refnum<vi>)  [unwired: 2 in, 1 out]
        n205 = for {
          tunnel: w468 -> [w478] mode=indexing
          shift-right: [w479] -> _
          shift-left: w467 -> [w480]
          tunnel: w466 -> [w477]
          tunnel: [w476] -> w465
          shift-right: [w474] -> w464
          shift-left: string[] [] -> [w473]
          n206 = call "getchildren.vi"("error in (no error)"=w477, "Parent Tag"=w478, "Tree Reference In"=w480) -> ("error out"=w476:errorcluster, "Children Tags"=w475:string[], "Tree Reference Out"=w479:refnum<vi>)
          n207 = Build Array (concatenate)(w473, w475) -> (w474:string[])
        }
        "Children Tags" <- w464
        n208 = call <vilib>:"Add State(s) to Queue__jki_lib_state_machine.vi"("State(s) in (\"\")"=w470) -> ("States Out"=w471:string)  [unwired: 14 in]
      }
      frame "UI: Cursor Set" {
        # "Argument"
        # "Set and Unset Cursor Busy.\n(Usage: \"UI: Cursor Set >> Busy|Idle\")"
        n209 = case shown="\"Idle\", Default" w481 {
          tunnel: w483 -> [w488 w490]
          tunnel: [w487 w489] -> w482
          frame "Idle", Default {
            n210 = call <vilib>:"Unset Busy.vi"("error in (no error)"=w488) -> ("error out"=w487:errorcluster)  [unwired: 10 in]
          }
          frame "Busy" {
            n211 = call <vilib>:"Set Busy.vi"("error in (no error)"=w490) -> ("error out"=w489:errorcluster)  [unwired: 9 in, 1 out]
          }
        }
        n212 = call <vilib>:"Add State(s) to Queue__jki_lib_state_machine.vi"("State(s) in (\"\")"=w486) -> ("States Out"=w485:string)  [unwired: 14 in]
      }
      frame "UI: Front Panel State" {
        # "Argument"
        # "Set Front Panel Open or Closed\n(Usage: \"UI: Front Panel State >> Open|Close\")"
        n213 = Unbundle By Name(w493) -> ("Core.Current VI Reference"=w492:refnum<vi>)
        n214 = case shown="\"Open\", Default" w491 {
          tunnel: w495 -> [w501 w514]
          tunnel: [w503 w515] -> w494
          tunnel: w492 -> [w502 w512]
          frame "Open", Default {
            n215 = property class="VI"(reference=w502, error in=w501) -> (reference out=w499:refnum<vi>, error out=w500:errorcluster, "Front Panel.Open"=w498:bool)
            n216 = case shown="False" w498 {
              tunnel: [w506 w509] -> w503
              tunnel: w500 -> [w505 w509]
              tunnel: w499 -> [w504 _]
              frame False {
                n217 = invoke class="VI" method="FP.Open"(reference=w504, error in=w505, "Activate"=TRUE, "State"=T9."Standard") -> (error out=w506:errorcluster)  [unwired: 1 in, 4 out]
              }
              frame True {
              }
            }
          }
          frame "Close" {
            n218 = property class="VI"(reference=w512, error in=w514) -> (reference out=w511:refnum<vi>, error out=w513:errorcluster, "Front Panel.Open"=w510:bool)
            n219 = case shown="True" w510 {
              tunnel: [w516 w519] -> w515
              tunnel: w513 -> [w516 w518]
              tunnel: w511 -> [_ w517]
              frame False {
              }
              frame True {
                n220 = invoke class="VI" method="FP.Close"(reference=w517, error in=w518) -> (error out=w519:errorcluster)  [unwired: 1 in, 2 out]
              }
            }
          }
        }
        n221 = call <vilib>:"Add State(s) to Queue__jki_lib_state_machine.vi"("State(s) in (\"\")"=w497) -> ("States Out"=w496:string)  [unwired: 14 in]
      }
      frame "---------- Macro ----------" {
        # "Do not put any code in this frame.\n(It is a separator no-op. You can make a copy of this frame to create a new Macro frame)"
        n222 = call <vilib>:"Add State(s) to Queue__jki_lib_state_machine.vi"("State(s) in (\"\")"=w523) -> ("States Out"=w522:string)  [unwired: 14 in]
      }
      frame "Macro: Initialize" {
        w524 = "Data: Initialize\nInitialize Core Data\nUI: Initialize\nUI: update presets\nUI: Front Panel State >> Open\nUI: Get Tree Items\nMISC: get preset from arguments"  # Data: Initialize Initialize Core Data UI: Initialize UI: update presets UI: Front Panel State >> Open UI: Get Tree Items MISC: get preset from arguments
        # "Initialization Macro\n(This is called once, when the VI starts)"
        n223 = call <vilib>:"Add State(s) to Queue__jki_lib_state_machine.vi"("State(s) in Front (\"\")"=w524, "State(s) in (\"\")"=w528) -> ("States Out"=w527:string)  [unwired: 13 in]
      }
      frame "Macro: Exit" {
        # "Exit Macro\n(This is called once, when the VI exits)"
        n224 = Unbundle By Name(w535) -> ("Core.Close Panel on Exit?"=w534:bool)
        n225 = Select(t="UI: Front Panel State >> Close", s=w534, f="") -> (s? t:f=w531:string)
        n226 = call <vilib>:"Add State(s) to Queue__jki_lib_state_machine.vi"("State(s) in (\"\")"=w531, "State(s) at Back (\"\")"="Data: Cleanup\nExit") -> ("States Out"=w529:string)  [unwired: 13 in]
        n227 = call <vilib>:"Add State(s) to Queue__jki_lib_state_machine.vi"("State(s) in Front (\"\")"=w529, "State(s) in (\"\")"=w538) -> ("States Out"=w537:string)  [unwired: 13 in]
      }
      frame "---------- Data Query ----------" {
        # "Template Separator\n(You can make a copy of, or modify, this frame)"
        n228 = call <vilib>:"Add State(s) to Queue__jki_lib_state_machine.vi"("State(s) in (\"\")"=w542) -> ("States Out"=w541:string)  [unwired: 14 in]
      }
      frame "----------------Traces----------------" {
        # "Template Separator\n(You can make a copy of, or modify, this frame)"
        n229 = call <vilib>:"Add State(s) to Queue__jki_lib_state_machine.vi"("State(s) in (\"\")"=w546) -> ("States Out"=w545:string)  [unwired: 14 in]
      }
      frame "MISC: get preset from arguments" {
        # "Template Separator\n(You can make a copy of, or modify, this frame)"
        n230 = disable-structure "Factory Pattern: Enable plugin" shown="RUN_TIME_ENGINE==True" {
          disable-tunnel: [_ ""] -> w547
          frame condition #0 (active) {
          }
          frame condition #1 {
            n231 = control-ref of="This Application"() -> (w559:refnum<vi>)
            n232 = property class="App"(reference=w559) -> ("App.Args"=w557:string[])  [unwired: 1 in, 2 out]
            n233 = Index Array(array=w557, index=1) -> (element=w554:string)
            "Argument" <- w554
            n234 = property on="Presets" class="Ring (strict)"() -> ("Strings []"=w555:string[])  [unwired: 2 in, 2 out]
            n235 = Search 1D Array(1D array=w555, element=w554) -> (index of element=w553:i32)  [unwired: 1 in]
            n236 = Greater Or Equal To 0?(x=w553) -> (x >= 0?=w552:bool)
            n237 = case shown="True" w552 {
              tunnel: w553 -> [_ w560]
              frame False {
              }
              frame True {
                n238 = property on="Presets" class="Ring (strict)"("Val(Sgnl)"=w560) -> ()  [unwired: 2 in, 2 out]
              }
            }
          }
        }
        n239 = call <vilib>:"Add State(s) to Queue__jki_lib_state_machine.vi"("State(s) in Front (\"\")"=w547, "State(s) in (\"\")"=w551) -> ("States Out"=w550:string)  [unwired: 13 in]
      }
      frame "Plot: Update Plot from Presets" {
        n240 = Unbundle By Name(w564) -> ("Traces"=w565:T2)
        n241 = for {
          tunnel: w565 -> [w570] mode=indexing
          tunnel: [w569] -> w561 mode=indexing
          n242 = Unbundle By Name(w570) -> ("Name"=w569:string)
        }
        n243 = property on="Tree" class="Tree (strict)"("Value"=w561) -> ()  [unwired: 2 in, 2 out]
        n244 = Bundle By Name(cluster=w564, "Trace Names"=w561) -> (w563:T10)
        n245 = call <vilib>:"Add State(s) to Queue__jki_lib_state_machine.vi"("State(s) in Front (\"\")"="Plot: Calculate interpolation interval>>preset" ("State(s) in Front (\"\")"), "State(s) in (\"\")"=w568) -> ("States Out"=w567:string)  [unwired: 13 in]
      }
      frame "Traces: update cluster" {
        # "Template Separator\n(You can make a copy of, or modify, this frame)"
        n246 = Unbundle By Name(w573) -> ("Traces"=w574:T2)
        n247 = for {
          tunnel: w574 -> [w581] mode=indexing
          tunnel: [w578] -> w571 mode=indexing
          i -> [w583]
          n248 = control-ref of="XY Graph"() -> (w584:refnum<vi>)
          n249 = property class="XYGraph (strict)"(reference=w584, "Active Plot"=w583) -> ("Plot.YScaleIdx"=w582:u32, "Plot.Plot Color"=w579:u32)  [unwired: 1 in, 2 out]
          n250 = Not Equal To 0?(x=w582) -> (x != 0?=w580:bool)
          n251 = Bundle By Name(cluster=w581, "L/R scale"=w580, "Color Box"=w579) -> (w578:T7)
        }
        n252 = Bundle By Name(cluster=w573, "Traces"=w571) -> (w572:T10)
        n253 = local write "Traces"(w571) -> ()
        n254 = call <vilib>:"Add State(s) to Queue__jki_lib_state_machine.vi"("State(s) in (\"\")"=w577) -> ("States Out"=w576:string)  [unwired: 14 in]
      }
      frame "Plot: Calculate interpolation interval" {
        n255 = Unbundle By Name(w593) -> ("time interval.stop timestamp (now)"=w595:timestamp, "time interval.start timestamp"=w594:timestamp, "max points per trace (all)"=w590:i32)
        n256 = To Double Precision Float(number=w595) -> (double precision float=w596:dbl)
        n257 = To Double Precision Float(number=w594) -> (double precision float=w597:dbl)
        n258 = Subtract(x=w596, y=w597) -> (x-y=w591:dbl)
        n259 = Divide(x=w591, y=w590) -> (x/y=w589:dbl)
        n260 = Format Into String(format string="Plot: Query Data>>%s", w587) -> (resulting string=w585:string)  [unwired: 2 in, 1 out]
        n261 = Round To Nearest(number=w589) -> (nearest integer value=w588:dbl)
        n262 = Bundle By Name(cluster=w593, "options.interpolation interval (1 s)"=w588) -> (w592:T10)
        n263 = call <vilib>:"Add State(s) to Queue__jki_lib_state_machine.vi"("State(s) in Front (\"\")"=w585, "State(s) in (\"\")"=w600) -> ("States Out"=w599:string)  [unwired: 13 in]
      }
      frame "Plot: Query Data" {
        n264 = Unbundle By Name(w616) -> ("max points per trace (all)"=w614:i32, "Trace Names"=w617:string[], "time interval"=w612:T5, "options"=w611:T1)
        n265 = property on="time interval" class="Clust (strict)"("Value"=w612) -> ()  [unwired: 2 in, 2 out]
        n266 = property on="options" class="Clust (strict)"("Value"=w611) -> ()  [unwired: 2 in, 2 out]
        n267 = Empty Array?(array=w617) -> (empty?=w618:bool)
        n268 = call <userlib>:"Tick Count (ms)__ogtk.vi"("error in (no error)"=w610) -> ("error out"=w609:errorcluster, "millisecond timer value"=w605:u32)  [unwired: 9 in]
        n269 = case shown="False" w618 {
          tunnel: w617 -> [w636 _]
          tunnel: w612 -> [w645 _]
          tunnel: w609 -> [w649 w734]
          tunnel: [w646 w734] -> w608
          tunnel: w611 -> [w644 _]
          tunnel: w616 -> [w648 w735]
          tunnel: [w647 w735] -> w615
          tunnel: w614 -> [w637 _]
          tunnel: [w630 _] -> w613
          tunnel: w601 -> [w631 _]
          frame False {
            (unwired) path "\\\\LASERBAY-DEV\\Belladata" ("database URL")
            (unwired) path "\\\\RPIX\\Belladata" ("database URL")
            n270 = First Call?() -> (First Call?: T/F=w641:bool)
            n271 = String To IP() -> (0:w622:u32[])  [unwired: 1 in]
            n272 = case shown="False" w641 {
              tunnel: [w725 30 ("timeout (30 s)")] -> w638
              tunnel: w636 -> [w731 _]
              frame False {
                n273 = Array Size(array=w731) -> (size(s)=w730:i32)
                n274 = Multiply(x=w730, y=3 ("timeout (30 s)")) -> (x*y=w728:i32)
                n275 = In Range and Coerce(upper limit=10, x=w728, lower limit=1) -> (coerced(x)=w725:i32)  [unwired: 1 out]
              }
              frame True {
              }
            }
            n276 = local read "empty?"() -> (w634:bool)
            n277 = Reverse 1D Array(array=w622) -> (reversed array=w623:u32[])
            n278 = for {
              tunnel: w623 -> [w650] mode=indexing
              tunnel: [w651] -> w626 mode=indexing
              n279 = IP To String(1:TRUE ("dot notation? (F)"), 2:w650) -> (0:w652:string)
              n280 = Match Pattern(string=w652, regular expression="192.168.") -> (after substring=w654:string)  [unwired: 1 in, 3 out]
              n281 = Match Pattern(string=w654, regular expression="\\.") -> (before substring=w651:string)  [unwired: 1 in, 3 out]
            }
            n282 = Search 1D Array(1D array=w626, element="10") -> (index of element=w628:i32)  [unwired: 1 in]
            n283 = Greater Or Equal To 0?(x=w628) -> (x >= 0?=w629:bool)
            n284 = Select(t=path "\\\\RPIX\\Belladata" ("Application Directory"), s=w629, f=path "\\\\LASERBAY-DEV\\Belladata" ("Application Directory")) -> (s? t:f=w621:path)
            n285 = case shown="True" w634 {
              tunnel: w621 -> [w657 w668]
              tunnel: w636 -> [_ w667]
              tunnel: w638 -> [_ w666]
              tunnel: w637 -> [_ w665]
              tunnel: [w657 w658] -> w633
              frame False {
              }
              frame True {
                n286 = Get Date/Time In Seconds() -> (seconds since 1Jan1904=w661:timestamp)
                n287 = To Double Precision Float(number=w661) -> (double precision float=w662:dbl)
                n288 = To Double Precision Float(number=w661) -> (double precision float=w664:dbl)
                n289 = Subtract(x=w662, y=900.0) -> (x-y=w671:dbl)
                n290 = Subtract(x=w664, y=30.0) -> (x-y=w660:dbl)
                n291 = To Time Stamp(1:w671) -> (0:w673:timestamp)
                n292 = To Time Stamp(1:w660) -> (0:w659:timestamp)
                n293 = local write "busy"(FALSE ("busy")) -> ()
                n294 = Bundle(w673, w659) -> (w669:cluster{timestamp, timestamp})  [unwired: 1 in]
                n295 = call-poly <vilib>:"Read Traces.vi"("timeout (30 s)"=w666, "max points per trace (all)"=w665, "time interval"=w669, "trace names"=w667, "database URL"=w668) -> ("database URL out"=w658:path)  [unwired: 3 in, 3 out]
              }
            }
            n296 = disable-structure shown="Enabled" {
              disable-tunnel: w636 -> [w685 w709]
              disable-tunnel: w633 -> [w684 w710]
              disable-tunnel: w645 -> [w683 w716]
              disable-tunnel: w644 -> [w682 w714]
              disable-tunnel: w637 -> [w681 w713]
              disable-tunnel: [w680 w707] -> w643
              disable-tunnel: [w678 w715] -> w642
              disable-tunnel: w638 -> [w677 w712]
              disable-tunnel: [w676 w711] -> w639
              disable-tunnel: [_ w706] -> w635
              frame Disabled {
                n297 = for {
                  tunnel: w685 -> [w693] mode=indexing
                  tunnel: w684 -> [w697]
                  tunnel: w683 -> [w695]
                  tunnel: w682 -> [w694]
                  tunnel: [w692] -> w676 mode=indexing
                  tunnel: [w691] -> w680 mode=indexing
                  tunnel: w681 -> [w686]
                  workers-P: 8 -> [_]
                  tunnel: [w690] -> w678
                  tunnel: w677 -> [w689]
                  tunnel: [w688] -> w674 mode=indexing
                  tunnel: [w687] -> w675 mode=indexing
                  n298 = disable-structure shown="Enabled" {
                    disable-tunnel: w697 -> [w704 w705]
                    disable-tunnel: [w702 _] -> w688
                    disable-tunnel: [w701 _] -> w687
                    disable-tunnel: [w700 w705] -> w696
                    disable-tunnel: w693 -> [w699 _]
                    frame Enabled {
                      n299 = call <vilib>:"Get Trace Info.vi"("timeout (30 s)"=5, "trace name"=w699, "database URL"=w704) -> ("error out"=w698:errorcluster, "last timestamp"=w701:timestamp, "first timestamp"=w702:timestamp, "database URL out"=w700:path)  [unwired: 4 in, 1 out]
                      n300 = call <vilib>:"Clear Errors.vi"("error in (no error)"=w698) -> ()  [unwired: 6 in, 1 out]
                    }
                    frame Disabled {
                    }
                  }
                  n301 = call-poly <vilib>:"Read Trace.vi"("options"=w694, "timeout (30 s)"=w689, "max points per trace (all)"=w686, "time interval"=w695, "trace name"=w693, "database URL"=w696) -> ("error out"=w690:errorcluster, "quality"=w691:i32[], "historical trace"=w692:cluster{"timestamps":timestamp[], "data":dbl[]})  [unwired: 2 in, 1 out]
                }
                "Array 2" <- w675
                "Array" <- w674
              }
              frame Enabled {
                n302 = disable-structure shown="Disabled" {
                  disable-tunnel: w710 -> [w719 _]
                  disable-tunnel: w709 -> [w718 _]
                  disable-tunnel: [w717 _] -> w708
                  frame Disabled {
                    n303 = for {
                      tunnel: w719 -> [w724]
                      tunnel: w718 -> [w722] mode=indexing
                      tunnel: [w721] -> w717
                      n304 = call <vilib>:"Get Trace Info.vi"("timeout (30 s)"=1, "trace name"=w722, "database URL"=w724) -> ("error out"=w721:errorcluster, "first timestamp"=w720:timestamp)  [unwired: 4 in, 3 out]
                      n305 = To Double Precision Float(number=w720) -> ()  [unwired: 1 out]
                    }
                  }
                  frame Enabled {
                  }
                }
                n306 = call-poly <vilib>:"Read Traces.vi"("options"=w714, "timeout (30 s)"=w712, "max points per trace (all)"=w713, "error in (no error)"=w708, "time interval"=w716, "trace names"=w709, "database URL"=w710) -> ("error out"=w715:errorcluster, "quality"=w707:i32[][], "historical traces"=w711:T6)  [unwired: 1 in, 1 out]
                n307 = Empty Array?(array=w707) -> (empty?=w706:bool)
              }
            }
            "quality" <- w643
            "error out" <- w642
            "empty?" <- w635
            n308 = Bundle By Name(cluster=w648, "historical traces"=w639) -> (w647:T10)
            n309 = Format Into String(format string="Plot: Display Data>>%s", w631) -> (resulting string=w630:string)  [unwired: 2 in, 1 out]
            n310 = for {
              tunnel: w642 -> [w733]
              tunnel: w639 -> [_] mode=indexing
              n311 = call <vilib>:"Clear Errors.vi"("error in (no error)"=w733) -> ()  [unwired: 6 in, 1 out]
            }
            n312 = call <vilib>:"Clear Errors.vi"("error in (no error)"=w649) -> ("error out"=w646:errorcluster)  [unwired: 6 in]
            "busy" <- TRUE ("Boolean")
          }
          frame True {
          }
        }
        n313 = call <userlib>:"Tick Count (ms)__ogtk.vi"("error in (no error)"=w608) -> ("error out"=w606:errorcluster, "millisecond timer value"=w607:u32)  [unwired: 9 in]
        n314 = Subtract(x=w607, y=w605) -> (x-y=w604:u32)
        n315 = Divide(x=w604, y=u32 1000 ("x")) -> (x/y=→"time (s)":dbl)
        n316 = call <vilib>:"Add State(s) to Queue__jki_lib_state_machine.vi"("State(s) in Front (\"\")"=w613, "State(s) in (\"\")"=w620) -> ("States Out"=w619:string)  [unwired: 13 in]
      }
      frame "Plot: Display Data" {
        n317 = Unbundle By Name(w742) -> ("historical traces"=→"XY Graph":T6, "Traces"=w737:T2)
        n318 = local write "busy"(FALSE ("Boolean")) -> ()
        n319 = case shown="\"preset\"" w738 {
          tunnel: w737 -> [_ w746]
          tunnel: ["Traces: update cluster" ("State(s) in Front (\"\")") "" ("State(s) in Front (\"\")")] -> w736
          frame "False", Default {
          }
          frame "preset" {
            n320 = for {
              tunnel: w746 -> [w751] mode=indexing
              i -> [w752]
              (unwired) u8 2 ("Y Scale.Scale Fit")
              n321 = control-ref of="XY Graph"() -> (w753:refnum<vi>)
              n322 = Unbundle By Name(w751) -> ("L/R scale"=w757:bool, "Color Box"=w750:u32)
              n323 = To Unsigned Long Integer(number=w752) -> (unsigned 32bit integer=w754:u32)
              n324 = Select(t=u32 1 ("f"), s=w757, f=u32 0) -> (s? t:f=w749:u32)
              n325 = property class="XYGraph (strict)"(reference=w753, "Active Plot"=w754, "Plot.YScaleIdx"=w749, "Plot.Plot Color"=w750, "ActYScl"=w749, "YScale.ScaleFit"=u8 2 ("Y Scale.Scale Fit")) -> ()  [unwired: 1 in, 2 out]
            }
          }
        }
        n326 = call <vilib>:"Add State(s) to Queue__jki_lib_state_machine.vi"("State(s) in Front (\"\")"=w736, "State(s) in (\"\")"=w744) -> ("States Out"=w743:string)  [unwired: 13 in]
      }
      frame "csv export" {
        n327 = Unbundle By Name(w759) -> ()  [unwired: 1 out]
        n328 = call <vilib>:"Add State(s) to Queue__jki_lib_state_machine.vi"("State(s) in (\"\")"=w761) -> ("States Out"=w760:string)  [unwired: 14 in]
      }
      frame "Plot: Display Current" {
        n329 = Get Date/Time In Seconds() -> (seconds since 1Jan1904=w768:timestamp)
        n330 = property on="Time slots" class="Enum (strict)"(error in=w765) -> (error out=w766:errorcluster, "Value"=w767:T4)  [unwired: 1 in, 1 out]
        n331 = property on="Time slots" class="Enum (strict)"(error in=w766, "Val(Sgnl)"=w767) -> (error out=w764:errorcluster)  [unwired: 1 in, 1 out]
        n332 = Bundle By Name(cluster=w770, "time interval.stop timestamp (now)"=w768, "Display Current Enable"=TRUE) -> (w769:T10)
        n333 = call <vilib>:"Add State(s) to Queue__jki_lib_state_machine.vi"("State(s) in Front (\"\")"="Plot: Calculate interpolation interval" ("State(s) in Front (\"\")"), "State(s) in (\"\")"=w772) -> ("States Out"=w771:string)  [unwired: 13 in]
      }
      frame "Plot: clear" {
        n334 = invoke on="Tree" class="Tree (strict)" method="Reinit To Default"(error in=w774) -> (error out=w773:errorcluster)  [unwired: 2 in, 2 out]
        n335 = property on="Time slots" class="Enum (strict)"(error in=w773) -> (error out=w779:errorcluster, "Value"=w780:T4)  [unwired: 1 in, 1 out]
        n336 = property on="Time slots" class="Enum (strict)"(error in=w779, "Val(Sgnl)"=w780) -> (error out=w778:errorcluster)  [unwired: 1 in, 1 out]
        n337 = Bundle By Name(cluster=w777, "Trace Names"=string[] []) -> (w776:T10)
        n338 = call <vilib>:"Add State(s) to Queue__jki_lib_state_machine.vi"("State(s) in (\"\")"=w782) -> ("States Out"=w781:string)  [unwired: 14 in]
      }
    }
  }
